vi "Node Archive and FTP File Handler ver2.vi"() -> ()   [LabVIEW 2010]
doc: "NODE ARCHIVE & FTP is a software used to handle the file management of remote field sites using the HTI Data Logger or ATR series acoustic equipment that generates *.RAT and *.ATL files. The software monitors a specific folder on the local machine that the HTI equipment has been set up to move completed files of these types into. All other file types are ignored. The software continues to scan this file until a new file is added to the directory, on the addition of a file the NODE ARCHIVE & FTP software moves the file into an Archive directory (and if specified into a redundant Archive directory) then creates a *.ZIP version of the file and retains a copy of it in the Archive directory as well. All Zip files are then copied to a specified FTP host.\n\nNODE ARCHIVE & FTP will not try and move files for the last five minutes of an hour, or for the first five to ten minutes of the hour (based on CPU time). This is to allow the HTI hardware time to move all files at the top of the hour and avoid conflict. During the rest of the hour the software will continue to scan for new files. At any time a user can force a scan or FTP move by selecting the Manual Force FTP button or the Manual Archive Files button.\n\nNODE ARCHIVE & FTP creates an .INI file and a .CSV file in the programs application directory. The .INI file retains the last values of the file directory and FTP credentials used. The .CSV retains a history of *.ZIP files moved to the FTP and the status of their move, if there were errors or not. NODE ARCHIVE & FTP will continue to try and send the file to the FTP host until that file has completed the process with no errors. DO NOT remove or edit the .CSV file or the software will try and move all files up to the FTP again and will slow down the FTP Host."
uses:
  FTP Credintials.ctl
  <vilib>/Utility/sysdir.llb/System Directory Type.ctl
  <vilib>/Utility/error.llb/DialogType.ctl
  <vilib>/Utility/config.llb/Read Key (String).vi
  <vilib>/Utility/config.llb/Read Key (Boolean).vi
  <vilib>/Utility/config.llb/Read Key (Path).vi
  <vilib>/Utility/config.llb/Read Key (I32).vi
  <vilib>/Utility/config.llb/Write Key (Path).vi
  <vilib>/Utility/config.llb/Write Key (String).vi
  <vilib>/Utility/config.llb/Write Key (I32).vi
  <vilib>/Utility/config.llb/Write Key (Boolean).vi
  <vilib>/Utility/config.llb/NI_LVConfig.lvlib
  Aarons labview builds/telemetryCode/Utilities/NewNI_SMTPEmail Folder/NewNI_SMTPEmail.lvlib
panel:
  in  "Time DaY":timestamp
  in  "Top level Tabs":T1(tab)
  in  "ShutDown":bool
  out "Status File move":bool caption="Archiving"
  out "Status FTP move":bool caption="FTP In Progress"
  in  "Manual FTP":bool
  in  "Manual Archive":bool
  in  "FTP Creds":T2 {"FTP Timeout (S)" min=0 max=300 step=1}
  in  "Archive Location 2":path caption="(Optional) External Directory To Archive *.RAT files"
  in  "Archive Location":path=path "C:/Archive" caption="Directory To Archive *.RAT files"
  in  "Rats Location":path=path "C:/Incoming" caption="Directory To Find *.RAT files"
  in  "Ping FTP Host":bool=TRUE
  in  "Ping Node 2":bool=TRUE
  in  "Ping Node 1":bool=TRUE
  out "Node 2 Response":bool
  in  "AddressNode2":string="www.google.com" caption="Address of Node 2 to Ping"
  out "FTP Response":bool
  out "Node1 Response":bool
  in  "recipients":string[](array[string])=["nmswyers@gmail.com"] caption="Email Recipients"
  in  "Addresshost":string="50.6.185.144" caption="Address of FTP host to Ping"
  in  "AddressNode 1":string="www.google.com" caption="Address of Node 1 to Ping"
  out "Elapsed Time (H)":dbl caption="Time to Next File \nSize Check (H)" format="%#_3f"
  out "Email Notification":T3 caption="Email Notification (From INI File)"
  # "DIRECTORY SETUP:"
  # "FTP SETUP:"
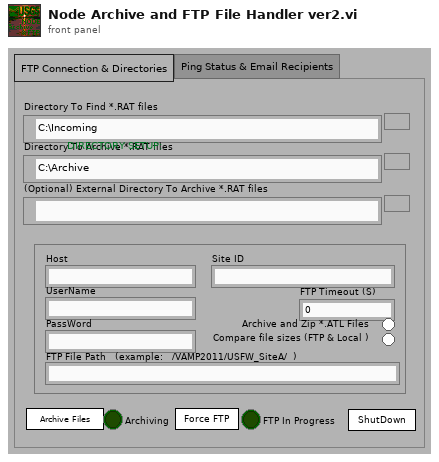
[diagram p1: front panel]
types:
  T1 = enum32{"FTP Connection & Directories", "Ping Status & Email Recipients"}
  T2 = typedef "FTP Credintials.ctl" = cluster{"Host":string, "UserName":string, "PassWord":string, "FTP File Path":string, "FTP Timeout (S)":i32, "Use ATL":bool, "Comp File Size":bool, "SITE ID":string, "Active or Passive":bool, "ASCII or Binary":bool}
  T3 = cluster{"Mail Server":string, "Return Address":string, "User Name":string, "Password":string}
  T4 = typedef "System Directory Type.ctl" = i32
  T5 = cluster{"Mail Server":string, "Return Address":string, "Email User Name":string, "Password":string}
  T6 = typedef "NI_LVConfig.lvlib/Config Data RefNum.ctl" = refnum<k1>
  T7 = typedef "DialogType.ctl" = u16
  T8 = cluster{"AddressNode 1":string, "AddressNode2":string, "Addresshost":string}
  T9 = enum16{"open", "replace", "create", "open or create", "replace or create", "replace or create with confirmation"}
  T10 = enum32{"invalid app kind", "Development System", "Run Time System", "Student Edition", "Embedded LabVIEW", "Evaluation", "Custom"}
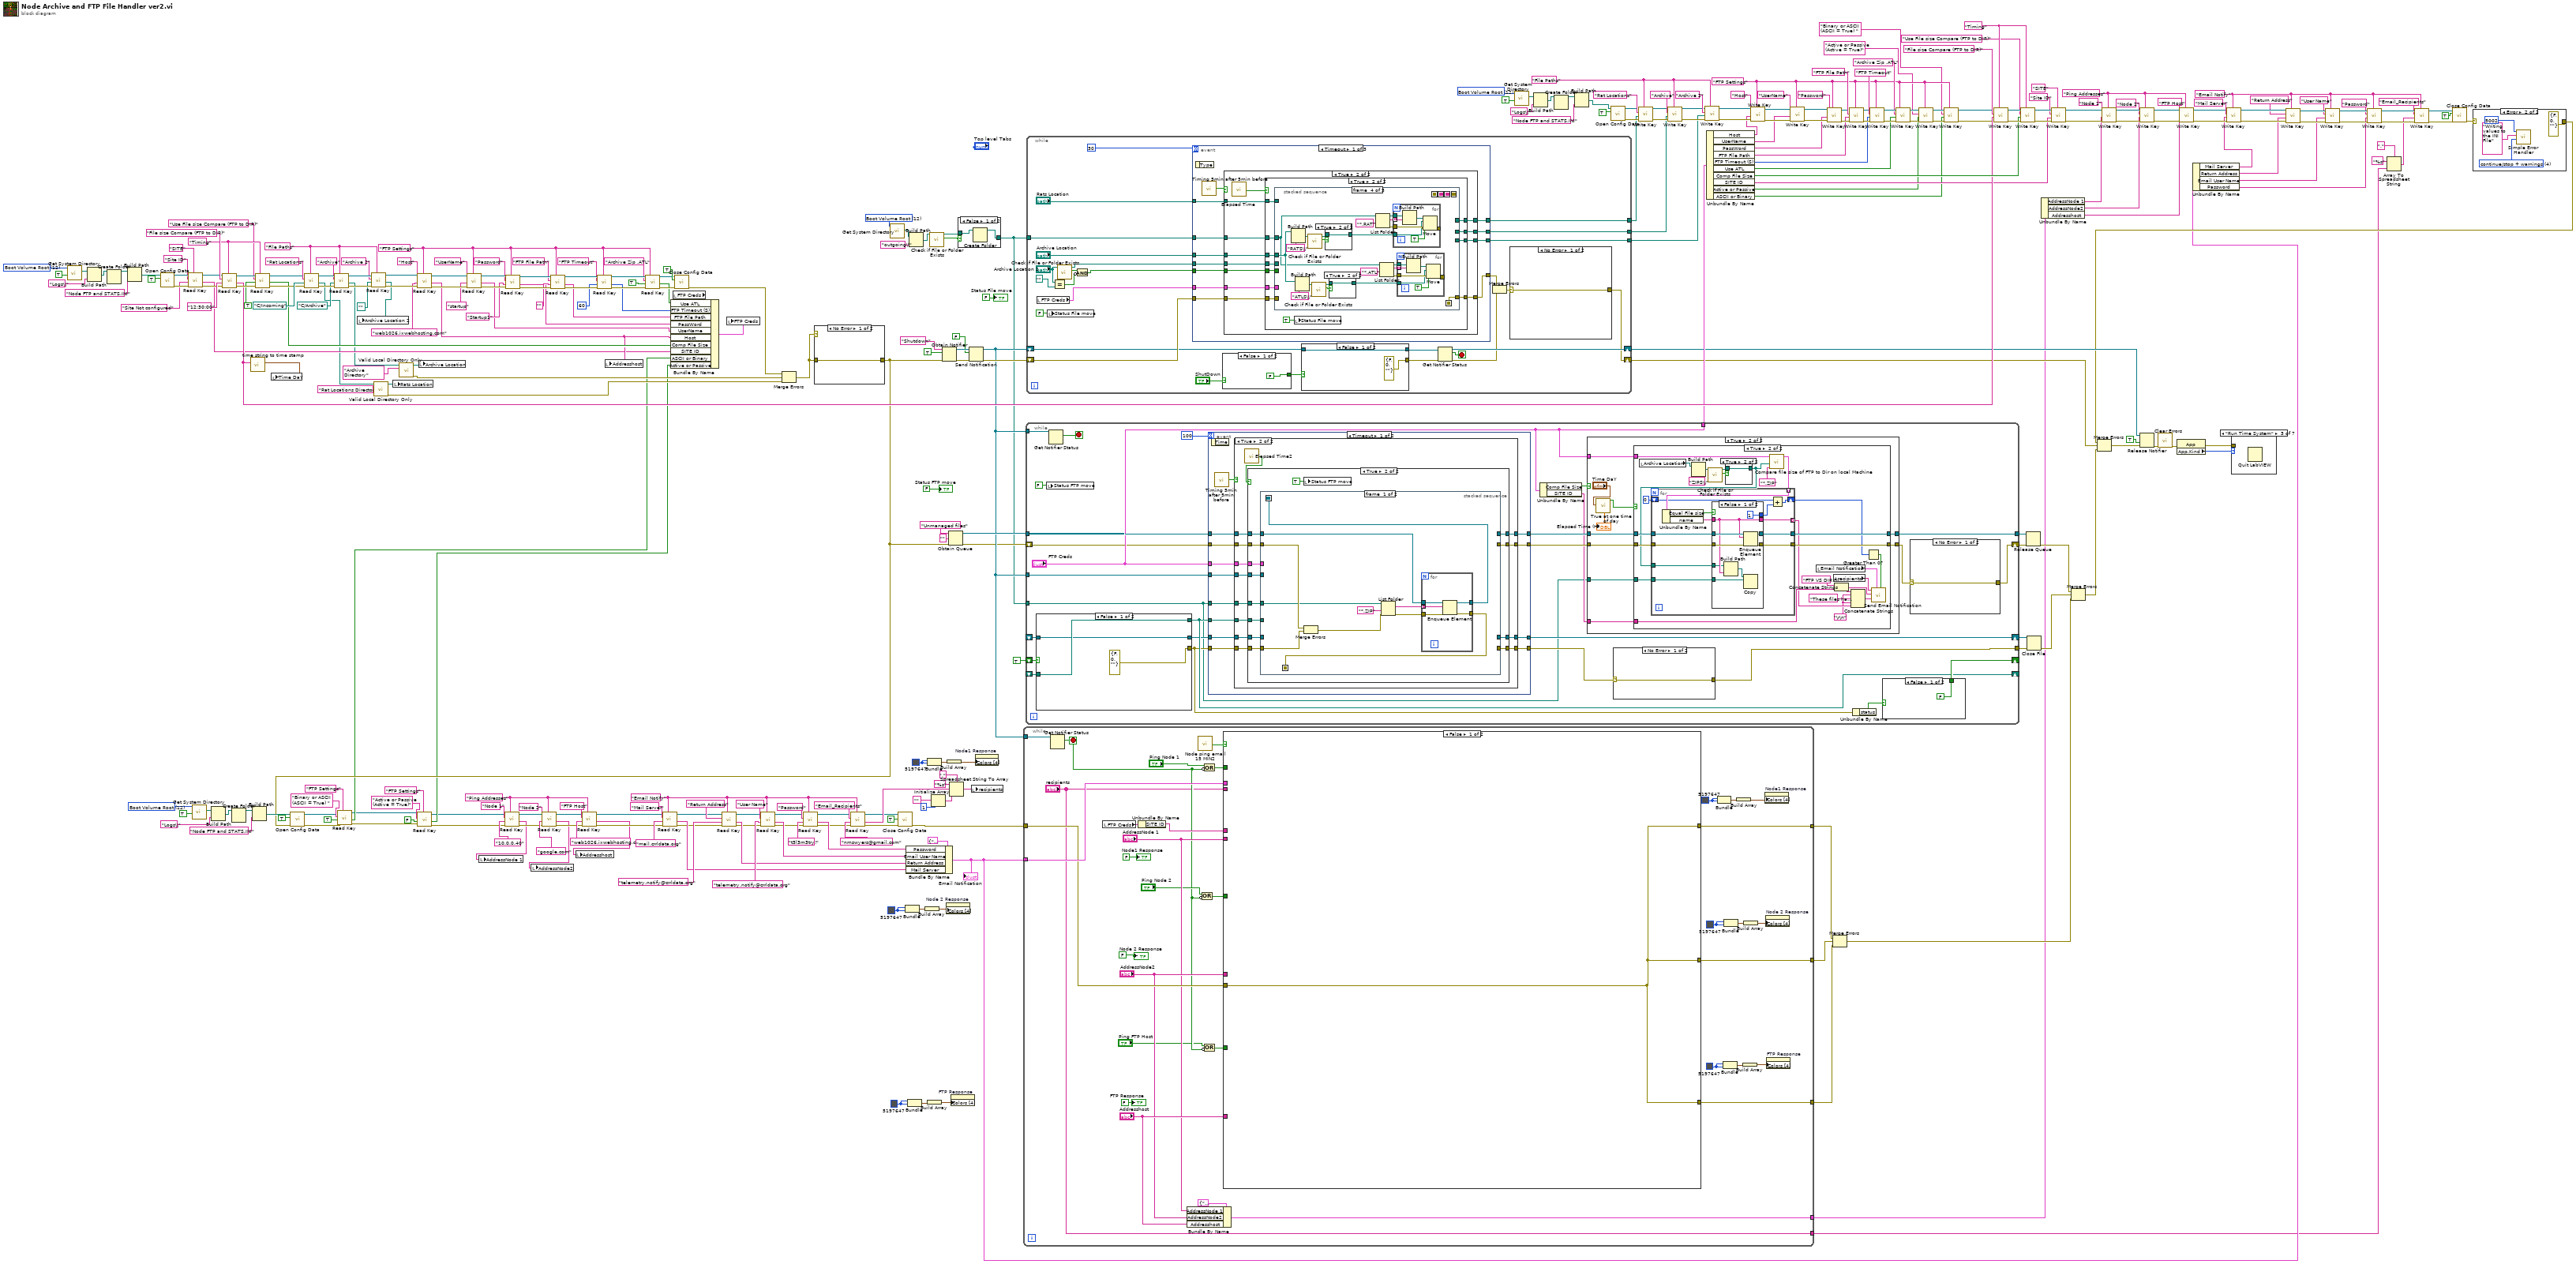
[diagram p0: block diagram]
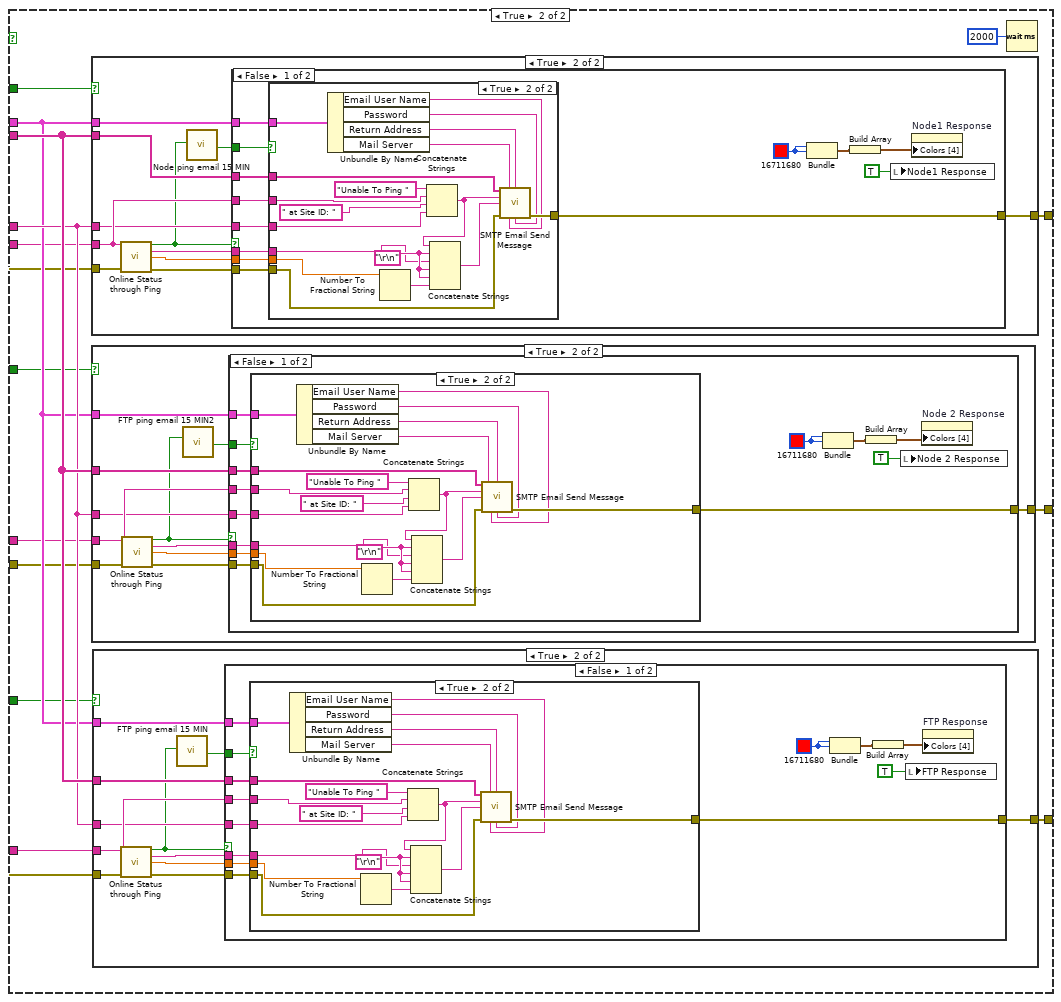
[diagram p3: hidden frame]
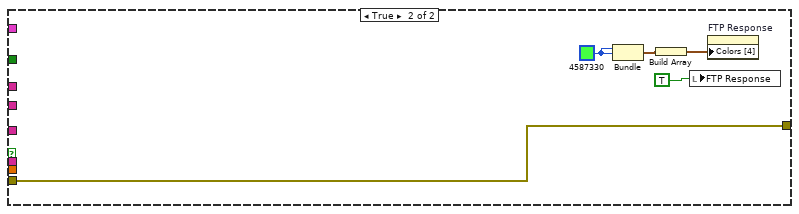
[diagram p6: hidden frame]
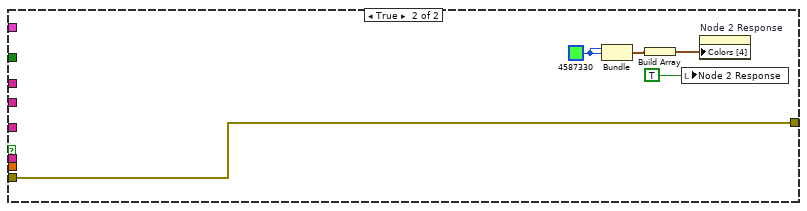
[diagram p9: hidden frame]
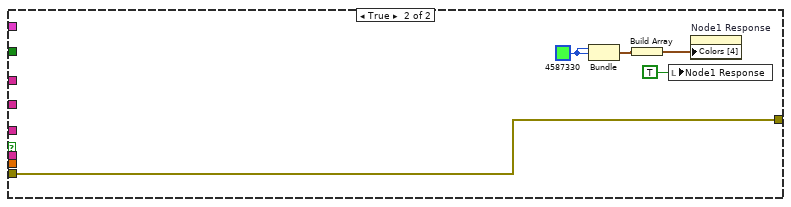
[diagram p12: hidden frame]
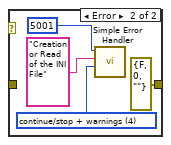
[diagram p14: hidden frame]
diagram:
  w21 = T4 12 items=["User Home"=0, "User Desktop"=1, "User Documents"=2, "User Application Data"=3, "User Preferences"=4, "User Temporary"=5, "Public Documents"=6, "Public Application Data"=7, "Public Preferences"=8, "Public Cache"=13, "System Core Libraries"=9, "System Installed Libraries"=10, "Application Files"=11, "Boot Volume Root"=12] ("system directory type")
  w26 = "Email Notify" ("name or relative path")
  w94 = "Ping Addresses" ("name or relative path")
  w107 = "Ping Addresses" ("name or relative path")
  w143 = u32 5197647 ("Color Box")
  w25 = "Email Notify" ("name or relative path")
  w153 = T4 12 items=["User Home"=0, "User Desktop"=1, "User Documents"=2, "User Application Data"=3, "User Preferences"=4, "User Temporary"=5, "Public Documents"=6, "Public Application Data"=7, "Public Preferences"=8, "Public Cache"=13, "System Core Libraries"=9, "System Installed Libraries"=10, "Application Files"=11, "Boot Volume Root"=12] ("system directory type")
  w169 = T4 12 items=["User Home"=0, "User Desktop"=1, "User Documents"=2, "User Application Data"=3, "User Preferences"=4, "User Temporary"=5, "Public Documents"=6, "Public Application Data"=7, "Public Preferences"=8, "Public Cache"=13, "System Core Libraries"=9, "System Installed Libraries"=10, "Application Files"=11, "Boot Volume Root"=12] ("system directory type")
  w207 = u32 5197647 ("Color Box")
  w204 = u32 5197647 ("Color Box")
  w215 = "Timing" ("name or relative path")
  w223 = "Timing" ("name or relative path")
  w7 = "FTP Settings" ("name or relative path")
  w262 = "File Paths" ("name or relative path")
  w297 = "FTP Settings" ("name or relative path")
  w315 = "File Paths" ("name or relative path")
  w317 = T4 12 items=["User Home"=0, "User Desktop"=1, "User Documents"=2, "User Application Data"=3, "User Preferences"=4, "User Temporary"=5, "Public Documents"=6, "Public Application Data"=7, "Public Preferences"=8, "Public Cache"=13, "System Core Libraries"=9, "System Installed Libraries"=10, "Application Files"=11, "Boot Volume Root"=12] ("system directory type")
  n1 = call <vilib>:"Get System Directory.vi"("create directory if not found? (F)"=TRUE, "system directory type"=w317) -> ("system directory"=w318:path)  [unwired: 9 in]
  n2 = Build Path(base path=w318, name or relative path="Logs\\" ("string")) -> (appended path=w179:path)
  n3 = Create Folder(path (use dialog)=w179) -> (created path=w178:path)  [unwired: 2 in, 2 out]
  n4 = Build Path(base path=w178, name or relative path="Node FTP and STATS.INI") -> (appended path=w176:path)
  n5 = call <vilib>:"Open Config Data.vi"("create file if necessary (T)"=TRUE, "configuration file path"=w176) -> ("error out"=w202:errorcluster, "refnum"=w201:T6)  [unwired: 7 in, 1 out]
  n6 = call-poly <vilib>:"Read Key.vi"("section"="SITE" ("name or relative path"), "error in (no error)"=w202, "default value"="Site Not configured", "key"="Site ID" ("name or relative path"), "refnum"=w201) -> ("error out"=w199:errorcluster, "value"=w195:string, "refnum out"=w200:T6)  [unwired: 3 in, 1 out]
  n7 = call <vilib>:"Get System Directory.vi"("create directory if not found? (F)"=TRUE, "system directory type"=w153) -> ("system directory"=w152:path)  [unwired: 9 in]
  n8 = Build Path(base path=w152, name or relative path="Logs\\" ("string")) -> (appended path=w158:path)
  n9 = call-poly <vilib>:"Read Key.vi"("section"=w223, "error in (no error)"=w199, "default value"="12:30:00", "key"="File size Compare (FTP to DIR)" ("name or relative path"), "refnum"=w200) -> ("error out"=w227:errorcluster, "value"=w210:string, "refnum out"=w226:T6)  [unwired: 3 in, 1 out]
  n10 = Create Folder(path (use dialog)=w158) -> (created path=w159:path)  [unwired: 2 in, 2 out]
  n11 = call "time string to time stamp.vi"("time string example(16:15:00)"=w210) -> ("time stamp"=w220:timestamp)  [unwired: 10 in]
  n12 = Build Path(base path=w159, name or relative path="Node FTP and STATS.INI") -> (appended path=w161:path)
  n13 = call-poly <vilib>:"Read Key.vi"("section"=w223, "error in (no error)"=w227, "default value"=TRUE ("create file if necessary (T)"), "key"="Use File size Compare (FTP to DIR)" ("name or relative path"), "refnum"=w226) -> ("error out"=w224:errorcluster, "value"=w212:bool, "refnum out"=w225:T6)  [unwired: 3 in, 1 out]
  n14 = local write "Time DaY"(w220) -> ()
  n15 = call-poly <vilib>:"Read Key.vi"("section"=w315, "error in (no error)"=w224, "default value"=path "C:/Incoming", "key"="Rat Locations" ("name or relative path"), "refnum"=w225) -> ("error out"=w322:errorcluster, "value"=w188:path, "refnum out"=w323:T6)  [unwired: 3 in, 1 out]
  n16 = call-poly <vilib>:"Read Key.vi"("section"=w315, "error in (no error)"=w322, "default value"=path "C:/Archive", "key"="Archive" ("name or relative path"), "refnum"=w323) -> ("error out"=w320:errorcluster, "value"=w184:path, "refnum out"=w321:T6)  [unwired: 3 in, 1 out]
  n17 = call-poly <vilib>:"Read Key.vi"("section"=w315, "error in (no error)"=w320, "default value"=path "", "key"="Archive 2" ("name or relative path"), "refnum"=w321) -> ("error out"=w311:errorcluster, "value"=w175:path, "refnum out"=w304:T6)  [unwired: 3 in, 1 out]
  n18 = local write "Archive Location 2"(w175) -> ()
  n19 = call "Valid Local Directory Only.vi"("Directory ref"="Rat Locations Directory", "Path input"=w188) -> ("error out"=w163:errorcluster, "Path output"=w186:path)  [unwired: 8 in]
  n20 = local write "Rats Location"(w186) -> ()
  n21 = call "Valid Local Directory Only.vi"("Directory ref"="Archive Directory", "Path input"=w184) -> ("error out"=w164:errorcluster, "Path output"=w183:path)  [unwired: 8 in]
  n22 = call-poly <vilib>:"Read Key.vi"("section"=w297, "error in (no error)"=w311, "default value"="web1026.ixwebhosting.com" ("name or relative path"), "key"="Host" ("name or relative path"), "refnum"=w304) -> ("error out"=w310:errorcluster, "value"=w208:string, "refnum out"=w303:T6)  [unwired: 3 in, 1 out]
  n23 = local write "Archive Location"(w183) -> ()
  n24 = call-poly <vilib>:"Read Key.vi"("section"=w297, "error in (no error)"=w310, "default value"="startup" ("name or relative path"), "key"="UserName" ("name or relative path"), "refnum"=w303) -> ("error out"=w309:errorcluster, "value"=w242:string, "refnum out"=w302:T6)  [unwired: 3 in, 1 out]
  n25 = call-poly <vilib>:"Read Key.vi"("section"=w297, "error in (no error)"=w309, "default value"="Startup1" ("name or relative path"), "key"="Password" ("name or relative path"), "refnum"=w302) -> ("error out"=w308:errorcluster, "value"=w243:string, "refnum out"=w301:T6)  [unwired: 3 in, 1 out]
  n26 = call-poly <vilib>:"Read Key.vi"("section"=w297, "error in (no error)"=w308, "default value"="" ("name or relative path"), "key"="FTP File Path" ("name or relative path"), "refnum"=w301) -> ("error out"=w307:errorcluster, "value"=w244:string, "refnum out"=w300:T6)  [unwired: 3 in, 1 out]
  n27 = call-poly <vilib>:"Read Key.vi"("section"=w297, "error in (no error)"=w307, "default value"=60, "key"="FTP Timeout" ("name or relative path"), "refnum"=w300) -> ("error out"=w306:errorcluster, "value"=w81:i32, "refnum out"=w299:T6)  [unwired: 3 in, 1 out]
  n28 = local write "Addresshost"(w208) -> ()
  n29 = call-poly <vilib>:"Read Key.vi"("section"=w297, "error in (no error)"=w306, "default value"=TRUE, "key"="Archive Zip .ATL" ("name or relative path"), "refnum"=w299) -> ("error out"=w305:errorcluster, "value"=w245:bool, "refnum out"=w298:T6)  [unwired: 3 in, 1 out]
  n30 = local read "FTP Creds"() -> (w246:T2)
  n31 = call <vilib>:"Close Config Data.vi"("error in (no error)"=w305, "write file if changed (T)"=TRUE, "refnum"=w298) -> ("error out"=w165:errorcluster)  [unwired: 7 in, 1 out]
  n32 = Merge Errors(w165, w164, w163) -> (w166:errorcluster)
  n33 = case shown="No Error" w166 {
    tunnel: w166 -> [w325 _]
    tunnel: [w325 errorcluster {"status"=FALSE, "code"=0, "source"=""} ("error out")] -> w118
    frame No Error {
    }
    frame Error {
      w329 = T7 4 items=["no dialog", "OK message", "continue or stop message", "OK message + warnings", "continue/stop + warnings"] ("type of dialog (OK msg:1)")
      n34 = call <vilib>:"Simple Error Handler.vi"("error code (no error:0)"=5001, "error source (\" \")"="Creation or Read of the INI File" ("error source (\" \")"), "type of dialog (OK msg:1)"=w329) -> ()  [unwired: 2 in, 5 out]
    }
  }
  n35 = call <vilib>:"Open Config Data.vi"("error in (no error)"=w118, "create file if necessary (T)"=TRUE, "configuration file path"=w161) -> ("error out"=w73:errorcluster, "refnum"=w74:T6)  [unwired: 6 in, 1 out]
  n36 = call-poly <vilib>:"Read Key.vi"("section"="FTP Settings" ("name or relative path"), "error in (no error)"=w73, "default value"=TRUE, "key"="Binary or ASCII (ASCII = True) " ("name or relative path"), "refnum"=w74) -> ("error out"=w14:errorcluster, "value"=w17:bool, "refnum out"=w15:T6)  [unwired: 3 in, 1 out]
  n37 = call-poly <vilib>:"Read Key.vi"("section"="FTP Settings" ("name or relative path"), "error in (no error)"=w14, "default value"=FALSE, "key"="Active or Passive (Active = True)" ("name or relative path"), "refnum"=w15) -> ("error out"=w12:errorcluster, "value"=w16:bool, "refnum out"=w13:T6)  [unwired: 3 in, 1 out]
  n38 = call-poly <vilib>:"Read Key.vi"("section"=w107, "error in (no error)"=w12, "default value"="10.0.0.40", "key"="Node 1" ("Mail Server"), "refnum"=w13) -> ("error out"=w105:errorcluster, "value"=w100:string, "refnum out"=w106:T6)  [unwired: 3 in, 1 out]
  n39 = local write "AddressNode 1"(w100) -> ()
  n40 = call-poly <vilib>:"Read Key.vi"("section"=w107, "error in (no error)"=w105, "default value"="google.com", "key"="Node 2" ("Mail Server"), "refnum"=w106) -> ("error out"=w104:errorcluster, "value"=w99:string, "refnum out"=w103:T6)  [unwired: 3 in, 1 out]
  n41 = local write "AddressNode2"(w99) -> ()
  n42 = call-poly <vilib>:"Read Key.vi"("section"=w107, "error in (no error)"=w104, "default value"="web1026.ixwebhosting.com", "key"="FTP Host" ("Mail Server"), "refnum"=w103) -> ("error out"=w101:errorcluster, "value"=w98:string, "refnum out"=w102:T6)  [unwired: 3 in, 1 out]
  n43 = local write "Addresshost"(w98) -> ()
  n44 = call-poly <vilib>:"Read Key.vi"("section"=w25, "error in (no error)"=w101, "default value"="mail.crrldata.org", "key"="Mail Server" ("Mail Server"), "refnum"=w102) -> ("error out"=w71:errorcluster, "value"=w132:string, "refnum out"=w70:T6)  [unwired: 3 in, 1 out]
  n45 = Bundle By Name(cluster=w246, "Use ATL"=w245, "FTP Timeout (S)"=w81, "FTP File Path"=w244, "PassWord"=w243, "UserName"=w242, "Host"=w208, "Comp File Size"=w212, "SITE ID"=w195, "ASCII or Binary"=w17, "Active or Passive"=w16) -> (w247:T2)
  n46 = call-poly <vilib>:"Read Key.vi"("section"=w25, "error in (no error)"=w71, "default value"="telemetry.notify@crrldata.org", "key"="Return Address" ("Return Address"), "refnum"=w70) -> ("error out"=w69:errorcluster, "value"=w133:string, "refnum out"=w66:T6)  [unwired: 3 in, 1 out]
  n47 = local write "FTP Creds"(w247) -> ()
  n48 = call-poly <vilib>:"Read Key.vi"("section"=w25, "error in (no error)"=w69, "default value"="telemetry.notify@crrldata.org", "key"="User Name" ("Email User Name"), "refnum"=w66) -> ("error out"=w68:errorcluster, "value"=w134:string, "refnum out"=w67:T6)  [unwired: 3 in, 1 out]
  n49 = call-poly <vilib>:"Read Key.vi"("section"=w25, "error in (no error)"=w68, "default value"="t3l3m3try!", "key"="Password" ("Password"), "refnum"=w67) -> ("error out"=w57:errorcluster, "value"=w135:string, "refnum out"=w58:T6)  [unwired: 3 in, 1 out]
  n50 = call-poly <vilib>:"Read Key.vi"("section"=w25, "error in (no error)"=w57, "default value"="nmswyers@gmail.com", "key"="Email_Recipients" ("Password"), "refnum"=w58) -> ("error out"=w54:errorcluster, "value"=w56:string, "refnum out"=w55:T6)  [unwired: 3 in, 1 out]
  n51 = call <vilib>:"Get System Directory.vi"("system directory type"=w21) -> ("system directory"=w22:path)  [unwired: 10 in]
  n52 = call <vilib>:"Close Config Data.vi"("error in (no error)"=w54, "write file if changed (T)"=TRUE, "refnum"=w55) -> ("error out"=w146:errorcluster)  [unwired: 7 in, 1 out]
  n53 = Bundle("Color Box"=w207, "Color Box"=w207) -> (w206:cluster{"Color Box":u32, "Color Box":u32})  [unwired: 1 in]
  n54 = Bundle By Name(cluster=T5 {"Mail Server"="Mail Server", "Return Address"="Return Address", "Email User Name"="User Name", "Password"="Password"} ("input cluster"), "Password"=w135, "Email User Name"=w134, "Return Address"=w133, "Mail Server"=w132) -> (w35:T5)
  "Email Notification" <- w35
  n55 = Bundle("Color Box"=w143, "Color Box"=w143) -> (w144:cluster{"Color Box":u32, "Color Box":u32})  [unwired: 1 in]
  n56 = Build Path(base path=w22, name or relative path="outgoing\\") -> (appended path=w19:path)
  n57 = Build Array(w206) -> (w142:cluster{"Color Box":u32, "Color Box":u32}[])
  n58 = Bundle("Color Box"=w204, "Color Box"=w204) -> (w203:cluster{"Color Box":u32, "Color Box":u32})  [unwired: 1 in]
  n59 = Build Array(w144) -> (w145:cluster{"Color Box":u32, "Color Box":u32}[])
  n60 = call <vilib>:"Check if File or Folder Exists.vi"("path"=w19) -> ("file or folder exists?"=w23:bool, "dup path"=w24:path)  [unwired: 8 in, 1 out]
  n61 = Initialize Array("", 1 ("dimension size")) -> (w65:string[])
  n62 = Obtain Notifier(name (unnamed)="Shutdown", notification data type=TRUE, error in (no error)=w118) -> (notifier out=w129:refnum<notifier>, error out=w127:errorcluster)  [unwired: 1 in, 1 out]
  n63 = property on="Node 2 Response" class="Bool (strict)"("Colors [4]"=w142) -> ()  [unwired: 2 in, 2 out]
  n64 = Build Array(w203) -> (w205:cluster{"Color Box":u32, "Color Box":u32}[])
  n65 = Obtain Queue(name (unnamed)="Unmanaged files", element data type="" ("name (unnamed)"), error in (no error)=w118) -> (queue out=w234:refnum<queue>, error out=w72:errorcluster)  [unwired: 2 in, 1 out]
  n66 = Spreadsheet String To Array(delimiter (Tab)=",", format string="%s", spreadsheet string=w56, array type (2D Dbl)=w65) -> (array=w53:string[])
  n67 = property on="FTP Response" class="Bool (strict)"("Colors [4]"=w145) -> ()  [unwired: 2 in, 2 out]
  n68 = case shown="False" w23 {
    tunnel: w24 -> [w331 w332]
    tunnel: [w330 w332] -> w18
    frame False {
      n69 = Create Folder(path (use dialog)=w331) -> (created path=w330:path)  [unwired: 2 in, 2 out]
    }
    frame True {
    }
  }
  n70 = Send Notification(notification=FALSE, notifier=w129, error in (no error)=w127) -> (notifier out=w82:refnum<notifier>, error out=w126:errorcluster)
  n71 = local write "recipients"(w53) -> ()
  n72 = property on="Node1 Response" class="Bool (strict)"("Colors [4]"=w205) -> ()  [unwired: 2 in, 2 out]
  n73 = while {
    tunnel: w146 -> [w356]
    tunnel: [w363] -> w182
    tunnel: w35 -> [w358]
    tunnel: [w360] -> w141
    tunnel: [w359] -> w140
    tunnel: w82 -> [w357]
    tunnel: [w351] -> w97
    tunnel: ["recipients"] -> w30
    stop <- w345 stop-if-true
    w337 = u32 5197647 ("Color Box")
    w338 = u32 5197647 ("Color Box")
    w342 = u32 5197647 ("Color Box")
    n74 = Get Notifier Status(notifier=w357) -> (current notification=w345:bool)  [unwired: 1 in, 4 out]
    n75 = local read "FTP Creds"() -> (w364:T2)
    n76 = Unbundle By Name(w364) -> ("SITE ID"=w361:string)
    n77 = Bundle By Name(cluster=T8 {"AddressNode 1"="www.google.com", "AddressNode2"="www.google.com", "Addresshost"="50.6.185.144"} ("input cluster"), "AddressNode 1"="AddressNode 1", "AddressNode2"="AddressNode2", "Addresshost"="Addresshost") -> (w351:T8)
    n78 = call "Node ping email 15 MIN2"() -> ("Time has Elapsed"=w334:bool)  [unwired: 12 in, 7 out]
    n79 = Compound Arithmetic op=OR("Ping Node 2", invert w345) -> (w348:bool)
    n80 = Compound Arithmetic op=OR("Ping Node 1", invert w345) -> (w350:bool)
    n81 = Compound Arithmetic op=OR("Ping FTP Host", invert w345) -> (w346:bool)
    n82 = case shown="False" w334 {
      tunnel: [w367 w381] -> w363
      tunnel: "recipients" -> [_ w380]
      tunnel: w361 -> [_ w379]
      tunnel: [w367 w378] -> w360
      tunnel: [w367 w377] -> w359
      tunnel: w358 -> [_ w376]
      tunnel: w356 -> [w367 w375]
      tunnel: "Addresshost" -> [_ w374]
      tunnel: "AddressNode2" -> [_ w373]
      tunnel: "AddressNode 1" -> [_ w372]
      tunnel: w350 -> [_ w371]
      tunnel: w348 -> [_ w370]
      tunnel: w346 -> [_ w369]
      frame False {
      }
      frame True {
        n83 = case shown="True" w371 {
          tunnel: w372 -> [_ w489]
          tunnel: [w480 w487] -> w381
          tunnel: w380 -> [_ w486]
          tunnel: w375 -> [w480 w485]
          tunnel: w379 -> [_ w484]
          tunnel: w376 -> [_ w483]
          frame False {
          }
          frame True {
            n84 = call "Online Status through Ping.vi"("AddressToPing"=w489, "error in (no error)"=w485) -> ("Connection?"=w481:bool, "Standard Output"=w491:string, "% Recieved"=w490:dbl, "error out"=w488:errorcluster)  [unwired: 9 in, 1 out]
            n85 = call "Node ping email 15 MIN"("Reset"=w481) -> ("Time has Elapsed"=w482:bool)  [unwired: 11 in, 7 out]
            n86 = case shown="False" w481 {
              tunnel: w491 -> [w504 _]
              tunnel: w490 -> [w503 _]
              tunnel: w486 -> [w502 _]
              tunnel: w489 -> [w501 _]
              tunnel: w484 -> [w496 _]
              tunnel: w488 -> [w495 w524]
              tunnel: [w494 w524] -> w487
              tunnel: w483 -> [w493 _]
              tunnel: w482 -> [w492 _]
              frame False {
                w499 = u32 16711680 ("Color Box")
                n87 = case shown="True" w492 {
                  tunnel: w504 -> [_ w515]
                  tunnel: w503 -> [_ w518]
                  tunnel: w502 -> [_ w517]
                  tunnel: w501 -> [_ w516]
                  tunnel: w496 -> [_ w513]
                  tunnel: w495 -> [w505 w512]
                  tunnel: [w505 w511] -> w494
                  tunnel: w493 -> [_ w510]
                  frame False {
                  }
                  frame True {
                    w522 = "\r\n"
                    n88 = Unbundle By Name(w510) -> ("Email User Name"=w506:string, "Password"=w507:string, "Return Address"=w508:string, "Mail Server"=w509:string)
                    n89 = Number To Fractional String(number=w518) -> (F-format string=w521:string)  [unwired: 3 in]
                    n90 = Concatenate Strings("Unable To Ping " ("subject ([No Subject])"), w516, " at Site ID: " ("string"), w513) -> (w520:string)
                    n91 = Concatenate Strings(w520, w522, w515, w522, w522, w521) -> (w519:string)
                    n92 = call "SMTP Email Send Message.vi"("recipients"=w517, "mail server"=w509, "return address"=w508, "subject ([No Subject])"=w520, "message"=w519, "error in (no error)"=w512, "username"=w506, "password"=w507) -> ("error out"=w511:errorcluster)  [unwired: 7 out]
                  }
                }
                n93 = Bundle("Color Box"=w499, "Color Box"=w499) -> (w498:cluster{"Color Box":u32, "Color Box":u32})  [unwired: 1 in]
                n94 = Build Array(w498) -> (w500:cluster{"Color Box":u32, "Color Box":u32}[])
                n95 = local write "Node1 Response"(TRUE ("Node Responding")) -> ()
                n96 = property on="Node1 Response" class="Bool (strict)"("Colors [4]"=w500) -> ()  [unwired: 2 in, 2 out]
              }
              frame True {
                w527 = u32 4587330 ("Color Box")
                n97 = Bundle("Color Box"=w527, "Color Box"=w527) -> (w528:cluster{"Color Box":u32, "Color Box":u32})  [unwired: 1 in]
                n98 = Build Array(w528) -> (w526:cluster{"Color Box":u32, "Color Box":u32}[])
                n99 = local write "Node1 Response"(TRUE ("Node Responding")) -> ()
                n100 = property on="Node1 Response" class="Bool (strict)"("Colors [4]"=w526) -> ()  [unwired: 2 in, 2 out]
              }
            }
          }
        }
        n101 = case shown="True" w370 {
          tunnel: w373 -> [_ w439]
          tunnel: w380 -> [_ w438]
          tunnel: w375 -> [w431 w437]
          tunnel: w379 -> [_ w436]
          tunnel: [w431 w435] -> w378
          tunnel: w376 -> [_ w434]
          frame False {
          }
          frame True {
            n102 = call "Online Status through Ping.vi"("AddressToPing"=w439, "error in (no error)"=w437) -> ("Connection?"=w432:bool, "Standard Output"=w441:string, "% Recieved"=w440:dbl, "error out"=w442:errorcluster)  [unwired: 9 in, 1 out]
            n103 = call "FTP ping email 15 MIN2"("Reset"=w432) -> ("Time has Elapsed"=w433:bool)  [unwired: 11 in, 7 out]
            n104 = case shown="False" w432 {
              tunnel: w441 -> [w455 _]
              tunnel: w440 -> [w454 _]
              tunnel: w438 -> [w453 _]
              tunnel: w439 -> [w452 _]
              tunnel: w436 -> [w449 _]
              tunnel: w442 -> [w448 w477]
              tunnel: [w447 w477] -> w435
              tunnel: w434 -> [w444 _]
              tunnel: w433 -> [w443 _]
              frame False {
                w451 = u32 16711680 ("Color Box")
                n105 = case shown="True" w443 {
                  tunnel: w455 -> [_ w466]
                  tunnel: w454 -> [_ w469]
                  tunnel: w453 -> [_ w468]
                  tunnel: w452 -> [_ w467]
                  tunnel: w449 -> [_ w464]
                  tunnel: w448 -> [w456 w463]
                  tunnel: [w456 w462] -> w447
                  tunnel: w444 -> [_ w461]
                  frame False {
                  }
                  frame True {
                    w473 = "\r\n"
                    n106 = Unbundle By Name(w461) -> ("Email User Name"=w457:string, "Password"=w458:string, "Return Address"=w459:string, "Mail Server"=w460:string)
                    n107 = Number To Fractional String(number=w469) -> (F-format string=w472:string)  [unwired: 3 in]
                    n108 = Concatenate Strings("Unable To Ping " ("subject ([No Subject])"), w467, " at Site ID: " ("string"), w464) -> (w471:string)
                    n109 = Concatenate Strings(w471, w473, w466, w473, w473, w472) -> (w470:string)
                    n110 = call "SMTP Email Send Message.vi"("recipients"=w468, "mail server"=w460, "return address"=w459, "subject ([No Subject])"=w471, "message"=w470, "error in (no error)"=w463, "username"=w457, "password"=w458) -> ("error out"=w462:errorcluster)  [unwired: 7 out]
                  }
                }
                n111 = Bundle("Color Box"=w451, "Color Box"=w451) -> (w450:cluster{"Color Box":u32, "Color Box":u32})  [unwired: 1 in]
                n112 = Build Array(w450) -> (w446:cluster{"Color Box":u32, "Color Box":u32}[])
                n113 = local write "Node 2 Response"(TRUE ("FTP Responding")) -> ()
                n114 = property on="Node 2 Response" class="Bool (strict)"("Colors [4]"=w446) -> ()  [unwired: 2 in, 2 out]
              }
              frame True {
                w479 = u32 4587330 ("Color Box")
                n115 = Bundle("Color Box"=w479, "Color Box"=w479) -> (w478:cluster{"Color Box":u32, "Color Box":u32})  [unwired: 1 in]
                n116 = Build Array(w478) -> (w476:cluster{"Color Box":u32, "Color Box":u32}[])
                n117 = local write "Node 2 Response"(TRUE) -> ()
                n118 = property on="Node 2 Response" class="Bool (strict)"("Colors [4]"=w476) -> ()  [unwired: 2 in, 2 out]
              }
            }
          }
        }
        n119 = case shown="True" w369 {
          tunnel: w374 -> [_ w393]
          tunnel: w380 -> [_ w389]
          tunnel: w375 -> [w382 w388]
          tunnel: w379 -> [_ w387]
          tunnel: [w382 w386] -> w377
          tunnel: w376 -> [_ w385]
          frame False {
          }
          frame True {
            n120 = call "Online Status through Ping.vi"("AddressToPing"=w393, "error in (no error)"=w388) -> ("Connection?"=w383:bool, "Standard Output"=w391:string, "% Recieved"=w392:dbl, "error out"=w390:errorcluster)  [unwired: 9 in, 1 out]
            n121 = call "FTP ping email 15 MIN"("Reset"=w383) -> ("Time has Elapsed"=w384:bool)  [unwired: 11 in, 7 out]
            n122 = case shown="False" w383 {
              tunnel: w391 -> [w406 _]
              tunnel: w392 -> [w405 _]
              tunnel: w389 -> [w404 _]
              tunnel: w393 -> [w403 _]
              tunnel: w387 -> [w398 _]
              tunnel: w390 -> [w397 w426]
              tunnel: [w396 w426] -> w386
              tunnel: w385 -> [w395 _]
              tunnel: w384 -> [w394 _]
              frame False {
                w402 = u32 16711680 ("Color Box")
                n123 = case shown="True" w394 {
                  tunnel: w406 -> [_ w417]
                  tunnel: w405 -> [_ w420]
                  tunnel: w404 -> [_ w419]
                  tunnel: w403 -> [_ w418]
                  tunnel: w398 -> [_ w415]
                  tunnel: w397 -> [w407 w414]
                  tunnel: [w407 w413] -> w396
                  tunnel: w395 -> [_ w412]
                  frame False {
                  }
                  frame True {
                    w424 = "\r\n"
                    n124 = Unbundle By Name(w412) -> ("Email User Name"=w408:string, "Password"=w409:string, "Return Address"=w410:string, "Mail Server"=w411:string)
                    n125 = Number To Fractional String(number=w420) -> (F-format string=w423:string)  [unwired: 3 in]
                    n126 = Concatenate Strings("Unable To Ping " ("subject ([No Subject])"), w418, " at Site ID: " ("string"), w415) -> (w422:string)
                    n127 = Concatenate Strings(w422, w424, w417, w424, w424, w423) -> (w421:string)
                    n128 = call "SMTP Email Send Message.vi"("recipients"=w419, "mail server"=w411, "return address"=w410, "subject ([No Subject])"=w422, "message"=w421, "error in (no error)"=w414, "username"=w408, "password"=w409) -> ("error out"=w413:errorcluster)  [unwired: 7 out]
                  }
                }
                n129 = Bundle("Color Box"=w402, "Color Box"=w402) -> (w401:cluster{"Color Box":u32, "Color Box":u32})  [unwired: 1 in]
                n130 = Build Array(w401) -> (w400:cluster{"Color Box":u32, "Color Box":u32}[])
                n131 = local write "FTP Response"(TRUE ("FTP Responding")) -> ()
                n132 = property on="FTP Response" class="Bool (strict)"("Colors [4]"=w400) -> ()  [unwired: 2 in, 2 out]
              }
              frame True {
                w429 = u32 4587330 ("Color Box")
                n133 = Bundle("Color Box"=w429, "Color Box"=w429) -> (w428:cluster{"Color Box":u32, "Color Box":u32})  [unwired: 1 in]
                n134 = Build Array(w428) -> (w427:cluster{"Color Box":u32, "Color Box":u32}[])
                n135 = local write "FTP Response"(TRUE) -> ()
                n136 = property on="FTP Response" class="Bool (strict)"("Colors [4]"=w427) -> ()  [unwired: 2 in, 2 out]
              }
            }
          }
        }
        n137 = Wait (ms)(milliseconds to wait=u32 2000) -> ()  [unwired: 1 out]
      }
    }
    n138 = Bundle("Color Box"=w342, "Color Box"=w342) -> (w343:cluster{"Color Box":u32, "Color Box":u32})  [unwired: 1 in]
    n139 = Bundle("Color Box"=w338, "Color Box"=w338) -> (w339:cluster{"Color Box":u32, "Color Box":u32})  [unwired: 1 in]
    n140 = Bundle("Color Box"=w337, "Color Box"=w337) -> (w336:cluster{"Color Box":u32, "Color Box":u32})  [unwired: 1 in]
    n141 = Build Array(w343) -> (w341:cluster{"Color Box":u32, "Color Box":u32}[])
    n142 = Build Array(w339) -> (w340:cluster{"Color Box":u32, "Color Box":u32}[])
    n143 = Build Array(w336) -> (w335:cluster{"Color Box":u32, "Color Box":u32}[])
    n144 = property on="Node1 Response" class="Bool (strict)"("Colors [4]"=w341) -> ()  [unwired: 2 in, 2 out]
    n145 = property on="Node 2 Response" class="Bool (strict)"("Colors [4]"=w335) -> ()  [unwired: 2 in, 2 out]
    n146 = property on="FTP Response" class="Bool (strict)"("Colors [4]"=w340) -> ()  [unwired: 2 in, 2 out]
    "Node1 Response" <- FALSE
    "FTP Response" <- FALSE ("FTP Responding")
    "Node 2 Response" <- FALSE ("FTP Responding")
  }
  n147 = while {
    tunnel: w234 -> [w553]
    tunnel: [w544] -> w218
    shift-right: [w548] -> _
    shift-left: TRUE ("create directory if not found? (F)") -> [w551]
    shift-right: [w554] -> w237
    shift-left: _ -> [w550]
    shift-right: [w547] -> _
    shift-left: _ -> [w546]
    tunnel: ["FTP Creds"] -> w189
    tunnel: w82 -> [w537]
    tunnel: [w531] -> w114
    shift-right: [w535] -> w115
    shift-left: w72 -> [w533]
    tunnel: w82 -> [w534]
    tunnel: w18 -> [w529]
    stop <- w536 stop-if-true
    n148 = case shown="False" w551 {
      tunnel: w550 -> [w646 _]
      tunnel: [errorcluster {"status"=FALSE, "code"=0, "source"=""} ("error out") w651] -> w538
      tunnel: [w647 w650] -> w547
      tunnel: w546 -> [w647 _]
      tunnel: [w646 w649] -> w539
      frame False {
      }
      frame True {
        w657 = T4 12 items=["User Home"=0, "User Desktop"=1, "User Documents"=2, "User Application Data"=3, "User Preferences"=4, "User Temporary"=5, "Public Documents"=6, "Public Application Data"=7, "Public Preferences"=8, "Public Cache"=13, "System Core Libraries"=9, "System Installed Libraries"=10, "Application Files"=11, "Boot Volume Root"=12] ("system directory type")
        n149 = call <vilib>:"Get System Directory.vi"("create directory if not found? (F)"=TRUE, "system directory type"=w657) -> ("system directory"=w658:path)  [unwired: 9 in]
        n150 = Build Path(base path=w658, name or relative path="Logs\\" ("string")) -> (appended path=w654:path)
        n151 = Create Folder(path (use dialog)=w654) -> (created path=w653:path)  [unwired: 2 in, 2 out]
        n152 = Build Path(base path=w653, name or relative path="FTP File Move Record.CSV") -> (appended path=w650:path)
        n153 = Open/Create/Replace File(file path (use dialog)=w650, operation (0:open)=T9."open or create", access (0:read/write)=enum16{"read/write", "read-only", "write-only"}."read/write") -> (refnum out=w661:refnum<file>, error out=w662:errorcluster)  [unwired: 3 in, 1 out]
        n154 = Set File Position(refnum=w661, from (0:start)=enum16{"start", "end", "current"}."end", error in=w662) -> (refnum out=w649:refnum<file>, error out=w651:errorcluster)  [unwired: 1 in]
      }
    }
    n155 = local write "Status FTP move"(FALSE ("Status FTP move")) -> ()
    n156 = Get Notifier Status(notifier=w537) -> (current notification=w536:bool)  [unwired: 1 in, 4 out]
    n157 = event shown="[0] Timeout" {
      selector: _ -> [_ _]
      dyn-events: _ -> [_ _]
      timeout: 100 -> [_ _]
      tunnel: [w676 w809] -> w554
      tunnel: w553 -> [w675 w808]
      tunnel: [w674 w807] -> w545
      tunnel: w533 -> [w673 w806]
      tunnel: [w672 w805] -> w543
      tunnel: [w671 w804] -> w532
      tunnel: w539 -> [w669 w803]
      tunnel: w538 -> [w668 w802]
      tunnel: w547 -> [w667 w801]
      tunnel: "FTP Creds" -> [w666 w800]
      tunnel: w534 -> [w665 w799]
      tunnel: w529 -> [w664 w798]
      event Timeout {
        n158 = event-data() -> ()  [unwired: 1 in, 1 out]
        n159 = call "Timing 5min after 5min before.vi"() -> ("Mid Hour"=w670:bool)  [unwired: 5 in]
        n160 = case shown="True" w670 {
          tunnel: [w678 w693] -> w676
          tunnel: w675 -> [w680 w692]
          tunnel: [w680 w691] -> w674
          tunnel: w673 -> [w679 w690]
          tunnel: [w679 w689] -> w672
          tunnel: [w677 w688] -> w671
          tunnel: w669 -> [w678 w686]
          tunnel: w668 -> [w677 w685]
          tunnel: w667 -> [_ w684]
          tunnel: w666 -> [_ w683]
          tunnel: w665 -> [_ w682]
          tunnel: w664 -> [_ w681]
          frame False {
          }
          frame True {
            n161 = call "Elapsed Time2"() -> ("Time has Elapsed"=w687:bool)  [unwired: 12 in, 7 out]
            n162 = case shown="True" w687 {
              tunnel: [w694 w710] -> w693
              tunnel: w692 -> [w697 w709]
              tunnel: [w697 w708] -> w691
              tunnel: w690 -> [w696 w707]
              tunnel: [w696 w706] -> w689
              tunnel: [w695 w705] -> w688
              tunnel: w686 -> [w694 w703]
              tunnel: w685 -> [w695 w702]
              tunnel: w684 -> [_ w701]
              tunnel: w683 -> [_ w700]
              tunnel: w682 -> [_ w699]
              tunnel: w681 -> [_ w698]
              frame False {
              }
              frame True {
                n163 = stacked-sequence {
                  seq-local: [w719 _] -> [_ w737]
                  seq-local: [w718 _] -> [_ w736]
                  tunnel: [_ w740] -> w710
                  tunnel: w709 -> [w720 _]
                  tunnel: [_ w738] -> w708
                  tunnel: w707 -> [w717 w733]
                  tunnel: [_ w731] -> w706
                  tunnel: [_ w730] -> w705
                  tunnel: w703 -> [_ w729]
                  tunnel: w702 -> [w716 _]
                  tunnel: w701 -> [_ _]
                  tunnel: w700 -> [_ w728]
                  tunnel: w699 -> [_ w727]
                  tunnel: w698 -> [w713 w726]
                  frame #0 {
                    n164 = Merge Errors(w717, w716) -> (w712:errorcluster)
                    n165 = List Folder(path=w713, pattern="*.ZIP", error in=w712) -> (filenames=w714:string[], error out=w711:errorcluster)  [unwired: 1 in, 2 out]
                    n166 = for {
                      tunnel: w720 -> [w725]
                      tunnel: [w724] -> w719
                      tunnel: [w723] -> w718
                      tunnel: w714 -> [w722] mode=indexing
                      tunnel: w711 -> [w721]
                      n167 = Enqueue Element(queue=w725, element=w722, error in (no error)=w721) -> (queue out=w723:refnum<queue>, error out=w724:errorcluster)  [unwired: 1 in, 1 out]
                    }
                  }
                  frame #1 {
                    n168 = Get Queue Status(queue=w736, error in (no error)=w733) -> (queue out=w735:refnum<queue>, error out=w732:errorcluster, # elements in queue=w734:i32)  [unwired: 1 in, 5 out]
                    n169 = local read "Archive Location"() -> (w739:path)
                    n170 = for {
                      N: w734 -> [_]
                      tunnel: [w759] -> w740
                      tunnel: w737 -> [w758]
                      tunnel: w739 -> [w744]
                      tunnel: w735 -> [w747]
                      tunnel: [w755] -> w738
                      tunnel: [w757] -> w730
                      tunnel: w732 -> [w746]
                      tunnel: [w752] -> w731
                      tunnel: w729 -> [w751]
                      tunnel: w728 -> [w750]
                      tunnel: w727 -> [w748]
                      tunnel: w726 -> [w743]
                      n171 = Get Notifier Status(notifier=w748) -> (current notification=w745:bool)  [unwired: 1 in, 4 out]
                      n172 = Dequeue Element(queue=w747, timeout in ms (-1)=5, error in (no error)=w746) -> (queue out=w756:refnum<queue>, element=w741:string, error out=w753:errorcluster)  [unwired: 1 out]
                      n173 = call "FTP Move_Status_Errors.vi"("Archived Path dir"=w743, "FTP input cluster"=w750, "Queue elements"=w741) -> ("concatenated string of Error"=w742:string, "ReQue element  errored"=w749:bool)  [unwired: 7 in]
                      n174 = case shown="False" w745 {
                        tunnel: [w773 w792] -> w759
                        tunnel: w758 -> [w772 w791]
                        tunnel: [w771 w791] -> w757
                        tunnel: w756 -> [w770 w796]
                        tunnel: [w769 w795] -> w755
                        tunnel: w753 -> [w768 w794]
                        tunnel: [w767 w793] -> w752
                        tunnel: w751 -> [w766 w792]
                        tunnel: w742 -> [w765 _]
                        tunnel: w749 -> [w764 _]
                        tunnel: w741 -> [w763 _]
                        tunnel: w744 -> [w762 _]
                        tunnel: w743 -> [w761 _]
                        tunnel: w741 -> [w760 _]
                        frame False {
                          n175 = case shown="False" w764 {
                            tunnel: w770 -> [w775 w787]
                            tunnel: w763 -> [_ _]
                            tunnel: [w775 w787] -> w769
                            tunnel: w768 -> [w774 w786]
                            tunnel: [w774 w786] -> w767
                            tunnel: w762 -> [_ w781]
                            tunnel: w761 -> [_ w780]
                            tunnel: w760 -> [_ w776]
                            frame False {
                            }
                            frame True {
                              n176 = Build Path(base path=w781, name or relative path="ZIPS\\") -> (appended path=w785:path)
                              n177 = call <vilib>:"Check if File or Folder Exists.vi"("path"=w785) -> ("file or folder exists?"=w784:bool, "dup path"=w783:path)  [unwired: 8 in, 1 out]
                              n178 = Build Path(base path=w780, name or relative path=w776) -> (appended path=w779:path)
                              n179 = case shown="False" w784 {
                                tunnel: w783 -> [w789 w790]
                                tunnel: [w788 w790] -> w777
                                frame False {
                                n180 = Create Folder(path (use dialog)=w789) -> (created path=w788:path)  [unwired: 2 in, 2 out]
                                }
                                frame True {
                                }
                              }
                              n181 = Build Path(base path=w777, name or relative path=w776) -> (appended path=w778:path)
                              n182 = Move(source path=w779, 10:w778) -> ()  [unwired: 3 in, 3 out]
                            }
                          }
                          n183 = Write to Text File(file (use dialog)=w766, text=w765, error in=w772) -> (refnum out=w773:refnum<file>, error out=w771:errorcluster)  [unwired: 1 in, 1 out]
                        }
                        frame True {
                          n184 = Flush Queue(queue=w796, error in (no error)=w794) -> (queue out=w795:refnum<queue>, error out=w793:errorcluster)  [unwired: 1 out]
                        }
                      }
                    }
                  }
                }
                n185 = local write "Status FTP move"(TRUE ("Status FTP move")) -> ()
              }
            }
          }
        }
      }
      event "Manual FTP": Value Change {
        n186 = event-data() -> ()  [unwired: 1 in, 1 out]
        n187 = stacked-sequence {
          seq-local: [w818 _] -> [_ w836]
          seq-local: [w817 _] -> [_ w835]
          tunnel: [_ w839] -> w809
          tunnel: w808 -> [w819 _]
          tunnel: [_ w837] -> w807
          tunnel: w806 -> [w816 w832]
          tunnel: [_ w830] -> w805
          tunnel: [_ w829] -> w804
          tunnel: w803 -> [_ w828]
          tunnel: w802 -> [w815 _]
          tunnel: w801 -> [_ _]
          tunnel: w800 -> [_ w827]
          tunnel: w799 -> [_ w826]
          tunnel: w798 -> [w812 w825]
          frame #0 {
            n188 = Merge Errors(w816, w815) -> (w811:errorcluster)
            n189 = List Folder(path=w812, pattern="*.ZIP", error in=w811) -> (filenames=w813:string[], error out=w810:errorcluster)  [unwired: 1 in, 2 out]
            n190 = for {
              tunnel: w819 -> [w824]
              tunnel: [w823] -> w818
              tunnel: [w822] -> w817
              tunnel: w813 -> [w821] mode=indexing
              tunnel: w810 -> [w820]
              n191 = Enqueue Element(queue=w824, element=w821, error in (no error)=w820) -> (queue out=w822:refnum<queue>, error out=w823:errorcluster)  [unwired: 1 in, 1 out]
            }
          }
          frame #1 {
            n192 = Get Queue Status(queue=w835, error in (no error)=w832) -> (queue out=w834:refnum<queue>, error out=w831:errorcluster, # elements in queue=w833:i32)  [unwired: 1 in, 5 out]
            n193 = local read "Archive Location"() -> (w838:path)
            n194 = for {
              N: w833 -> [_]
              tunnel: [w858] -> w839
              tunnel: w836 -> [w857]
              tunnel: w838 -> [w843]
              tunnel: w834 -> [w846]
              tunnel: [w854] -> w837
              tunnel: [w856] -> w829
              tunnel: w831 -> [w845]
              tunnel: [w851] -> w830
              tunnel: w828 -> [w850]
              tunnel: w827 -> [w849]
              tunnel: w826 -> [w847]
              tunnel: w825 -> [w842]
              n195 = Get Notifier Status(notifier=w847) -> (current notification=w844:bool)  [unwired: 1 in, 4 out]
              n196 = Dequeue Element(queue=w846, timeout in ms (-1)=5, error in (no error)=w845) -> (queue out=w855:refnum<queue>, element=w840:string, error out=w852:errorcluster)  [unwired: 1 out]
              n197 = call "FTP Move_Status_Errors.vi"("Archived Path dir"=w842, "FTP input cluster"=w849, "Queue elements"=w840) -> ("concatenated string of Error"=w841:string, "ReQue element  errored"=w848:bool)  [unwired: 7 in]
              n198 = case shown="False" w844 {
                tunnel: [w872 w895] -> w858
                tunnel: w857 -> [w871 w894]
                tunnel: [w870 w894] -> w856
                tunnel: w855 -> [w869 w899]
                tunnel: [w868 w898] -> w854
                tunnel: w852 -> [w867 w897]
                tunnel: [w866 w896] -> w851
                tunnel: w850 -> [w865 w895]
                tunnel: w841 -> [w864 _]
                tunnel: w848 -> [w863 _]
                tunnel: w840 -> [w862 _]
                tunnel: w843 -> [w861 _]
                tunnel: w842 -> [w860 _]
                tunnel: w840 -> [w859 _]
                frame False {
                  n199 = case shown="True" w863 {
                    tunnel: w869 -> [w878 w890]
                    tunnel: w862 -> [w877 _]
                    tunnel: [w876 w890] -> w868
                    tunnel: w867 -> [w874 w889]
                    tunnel: [w873 w889] -> w866
                    tunnel: w861 -> [_ w884]
                    tunnel: w860 -> [_ w883]
                    tunnel: w859 -> [_ w879]
                    frame False {
                      n200 = Enqueue Element(queue=w878, element=w877, timeout in ms (-1)=5, error in (no error)=w874) -> (queue out=w876:refnum<queue>, error out=w873:errorcluster)  [unwired: 1 out]
                    }
                    frame True {
                      n201 = Build Path(base path=w884, name or relative path="ZIPS\\") -> (appended path=w888:path)
                      n202 = call <vilib>:"Check if File or Folder Exists.vi"("path"=w888) -> ("file or folder exists?"=w887:bool, "dup path"=w886:path)  [unwired: 8 in, 1 out]
                      n203 = Build Path(base path=w883, name or relative path=w879) -> (appended path=w882:path)
                      n204 = case shown="False" w887 {
                        tunnel: w886 -> [w892 w893]
                        tunnel: [w891 w893] -> w880
                        frame False {
                          n205 = Create Folder(path (use dialog)=w892) -> (created path=w891:path)  [unwired: 2 in, 2 out]
                        }
                        frame True {
                        }
                      }
                      n206 = Build Path(base path=w880, name or relative path=w879) -> (appended path=w881:path)
                      n207 = Move(source path=w882, 10:w881) -> ()  [unwired: 3 in, 3 out]
                    }
                  }
                  n208 = Write to Text File(file (use dialog)=w865, text=w864, error in=w871) -> (refnum out=w872:refnum<file>, error out=w870:errorcluster)  [unwired: 1 in, 1 out]
                }
                frame True {
                  n209 = Flush Queue(queue=w899, error in (no error)=w897) -> (queue out=w898:refnum<queue>, error out=w896:errorcluster)  [unwired: 1 out]
                }
              }
            }
          }
        }
        n210 = local write "Status FTP move"(TRUE ("Status FTP move")) -> ()
      }
    }
    n211 = Unbundle By Name("FTP Creds") -> ("Comp File Size"=w542:bool, "SITE ID"=w540:string)
    n212 = case shown="True" w542 {
      tunnel: w545 -> [w575 w583]
      tunnel: [w575 w582] -> w544
      tunnel: w543 -> [w574 w580]
      tunnel: [w574 w581] -> w530
      tunnel: "FTP Creds" -> [_ w579]
      tunnel: w540 -> [_ w577]
      tunnel: w529 -> [_ w576]
      frame False {
      }
      frame True {
        n213 = call "True at one time of day.vi"("Time stamp from INI (only will use time Not date)"="Time DaY") -> ("Time Until Next Scan (H)"=→"Elapsed Time (H)":dbl, "Time has Elapsed"=w584:bool)  [unwired: 8 in, 1 out]
        n214 = case shown="True" w584 {
          tunnel: w583 -> [w587 w609]
          tunnel: [w587 w611] -> w582
          tunnel: [w586 w610] -> w581
          tunnel: w580 -> [w586 w608]
          tunnel: w579 -> [_ w613]
          tunnel: w577 -> [_ w605]
          tunnel: w576 -> [_ w590]
          frame False {
          }
          frame True {
            w601 = "\r\n"
            n215 = local read "Archive Location"() -> (w591:path)
            n216 = Build Path(base path=w591, name or relative path="ZIPS\\") -> (appended path=w592:path)
            n217 = call <vilib>:"Check if File or Folder Exists.vi"("path"=w592) -> ("file or folder exists?"=w593:bool, "dup path"=w594:path)  [unwired: 8 in, 1 out]
            n218 = case shown="True" w593 {
              tunnel: w594 -> [w615 w616]
              tunnel: [w614 w616] -> w589
              frame False {
                n219 = Create Folder(path (use dialog)=w615) -> (created path=w614:path)  [unwired: 2 in, 2 out]
              }
              frame True {
              }
            }
            n220 = call "Compare file size of FTP to Dir on local Machine.vi"("File Pattern (*.CSV .ddf)"="*.ZIP", "Local Path to compare file sizes to FTP"=w589, "FTP Creds"=w613) -> ("Equal File Sizes"=w607:cluster{"name":string, "Equal File size":bool}[])  [unwired: 7 in, 1 out]
            n221 = for {
              tunnel: [w629] -> w611
              tunnel: [w628] -> w610
              tunnel: w609 -> [w626]
              tunnel: w608 -> [w627]
              tunnel: w607 -> [w625] mode=indexing
              tunnel: [w622] -> w604 mode=indexing
              shift-right: [w620] -> w606
              shift-left: 0 -> [w619]
              tunnel: w590 -> [w618]
              tunnel: w589 -> [w617]
              n222 = Unbundle By Name(w625) -> ("Equal File size"=w624:bool, "name"=w623:string)
              n223 = case shown="False" w624 {
                tunnel: [w638 w642] -> w629
                tunnel: [w637 w641] -> w628
                tunnel: w627 -> [w636 w641]
                tunnel: w626 -> [w635 w642]
                tunnel: w623 -> [w631 _]
                tunnel: [1 0] -> w621
                tunnel: [w631 ""] -> w622
                tunnel: w618 -> [w633 _]
                tunnel: w617 -> [w630 _]
                frame False {
                  n224 = Build Path(base path=w630, name or relative path=w631) -> (appended path=w632:path)
                  n225 = Copy(10:w633, 11:w632) -> ()  [unwired: 3 in, 3 out]
                  n226 = Enqueue Element(queue=w635, element=w631, error in (no error)=w636) -> (queue out=w638:refnum<queue>, error out=w637:errorcluster)  [unwired: 1 in, 1 out]
                }
                frame True {
                }
              }
              n227 = Add(x=w619, y=w621) -> (x+y=w620:i32)
            }
            n228 = local read "Email Notification"() -> (w596:T3)
            n229 = local read "recipients"() -> (w599:string[])
            n230 = Concatenate Strings("FTP VS DIR File sizes are different at Site ID: " ("string"), w605) -> (w598:string)
            n231 = Concatenate Strings(w598, w601, "These files have been re-queued for FTP move agian, check to make sure files are up to date and moving correctly.\nFiles of issue are listed below.\n\nLIST:" ("string"), w601, w604) -> (w597:string)
            n232 = Greater Than 0?(x=w606) -> (x > 0?=w600:bool)
            n233 = call "Send Email Notification.vi"("Send Email Notification"=w600, "Mail Creds"=w596, "message"=w597, "Email Subject"=w598, "recipients"=w599) -> ()  [unwired: 7 in]
          }
        }
      }
    }
    n234 = case shown="No Error" w532 {
      selector: w532 -> [w556 _]
      tunnel: [w556 errorcluster {"status"=FALSE, "code"=0, "source"=""} ("error IO")] -> w531
      frame No Error {
      }
      frame Error {
        n235 = local read "FTP Creds"() -> (w560:T2)
        n236 = Unbundle By Name(w560) -> ("SITE ID"=w559:string)
        n237 = local read "Email Notification"() -> (w562:T3)
        n238 = local read "recipients"() -> (w563:string[])
        n239 = Concatenate Strings("The Software was unable to write to the FTP Log at site ID: " ("Email Subject"), w559) -> (w557:string)
        n240 = call "Send Email Notification.vi"("Send Email Notification"=TRUE, "Mail Creds"=w562, "message"=w557, "Email Subject"=w557, "recipients"=w563) -> ()  [unwired: 7 in]
      }
    }
    n241 = Unbundle By Name(w538) -> ("status"=w549:bool)
    n242 = case shown="False" w549 {
      tunnel: [FALSE ("create directory if not found? (F)") TRUE ("create directory if not found? (F)")] -> w548
      frame False {
      }
      frame True {
        n243 = One Button Dialog(message="The File \"FTP FILE MOVE RECORD.CSV\" is open.\nPlease close the file before continuing.\n\nThis file is the log of past FTP movement and is needed by the software to maintain a history of already moved file. Please do not move or delete this file. This will result in unwanted actions by the software in attempt to send all files back up to the ftp again.\n") -> ()  [unwired: 1 in, 1 out]
      }
    }
    n244 = case shown="No Error" w530 {
      selector: w530 -> [w565 _]
      tunnel: [w565 errorcluster {"status"=FALSE, "code"=0, "source"=""} ("error IO")] -> w535
      frame No Error {
      }
      frame Error {
        n245 = local read "Email Notification"() -> (w571:T3)
        n246 = local read "recipients"() -> (w572:string[])
        n247 = local read "FTP Creds"() -> (w569:T2)
        n248 = Unbundle By Name(w569) -> ("SITE ID"=w568:string)
        n249 = Concatenate Strings("There was an Error with the FTP scan and Move at Site ID: " ("Email Subject"), w568) -> (w566:string)
        n250 = call "Send Email Notification.vi"("Send Email Notification"=TRUE, "Mail Creds"=w571, "message"=w566, "Email Subject"=w566, "recipients"=w572) -> ()  [unwired: 7 in]
      }
    }
  }
  n251 = while {
    shift-right: [w901] -> w125
    shift-left: w126 -> [w918]
    shift-right: [w906] -> w120
    shift-left: w82 -> [w909]
    tunnel: [w916] -> w240
    tunnel: [w915] -> w239
    tunnel: [w914] -> w238
    tunnel: w18 -> [w900]
    stop <- w907 stop-if-true
    n252 = local read "FTP Creds"() -> (w913:T2)
    n253 = local write "Status File move"(FALSE ("Status File move")) -> ()
    n254 = Equal?(x="Archive Location 2", y=path "") -> (x = y?=w926:bool)
    n255 = call <vilib>:"Check if File or Folder Exists.vi"("path"="Archive Location 2") -> ("file or folder exists?"=w925:bool, "dup path"=w921:path)  [unwired: 8 in, 1 out]
    n256 = Compound Arithmetic op=AND(w925, invert w926) -> (w922:bool)
    n257 = event shown="[0] Timeout" {
      selector: _ -> [_ _ _]
      dyn-events: _ -> [_ _ _]
      timeout: 30 -> [_ _ _]
      tunnel: w913 -> [w957 w1085 _]
      tunnel: w922 -> [w956 w1084 _]
      tunnel: w921 -> [w955 w1083 w1174]
      tunnel: "Archive Location" -> [w954 w1082 w1175]
      tunnel: "Rats Location" -> [w953 w1081 w1176]
      tunnel: w918 -> [w952 w1080 w1172]
      tunnel: [w951 w1079 w1171] -> w904
      tunnel: [w950 w1078 w1176] -> w916
      tunnel: [w949 w1077 w1175] -> w915
      tunnel: [w948 w1076 w1174] -> w914
      tunnel: w900 -> [w946 w1075 _]
      event Timeout {
        n258 = event-data() -> ()  [unwired: 1 in, 1 out]
        n259 = call "Timing 5min after 5min before.vi"() -> ("Mid Hour"=w947:bool)  [unwired: 5 in]
        n260 = case shown="True" w947 {
          tunnel: w953 -> [w961 w973]
          tunnel: w954 -> [w960 w972]
          tunnel: w955 -> [w959 w971]
          tunnel: w956 -> [_ w970]
          tunnel: w957 -> [_ w968]
          tunnel: [w961 w967] -> w950
          tunnel: [w960 w966] -> w949
          tunnel: [w959 w965] -> w948
          tunnel: w952 -> [w958 w964]
          tunnel: [w958 w963] -> w951
          tunnel: w946 -> [_ w962]
          frame False {
          }
          frame True {
            n261 = call "Elapsed Time"() -> ("Time has Elapsed"=w969:bool)  [unwired: 12 in, 7 out]
            n262 = case shown="True" w969 {
              tunnel: w973 -> [w977 w989]
              tunnel: w972 -> [w976 w988]
              tunnel: w971 -> [w975 w987]
              tunnel: w970 -> [_ w986]
              tunnel: w968 -> [_ w985]
              tunnel: [w977 w980] -> w967
              tunnel: [w976 w979] -> w966
              tunnel: [w975 w978] -> w965
              tunnel: w964 -> [w974 w984]
              tunnel: [w974 w983] -> w963
              tunnel: w962 -> [_ w981]
              frame False {
              }
              frame True {
                n263 = stacked-sequence {
                  seq-local: [_ w1003 _ _ _] -> [_ _ w1016 _ _]
                  seq-local: [w997 _ _ _ _] -> [_ w1009 _ _ _]
                  seq-local: [w996 _ _ _ _] -> [_ w1002 _ _ _]
                  seq-local: [_ w1006 _ _ _] -> [_ _ w1015 _ _]
                  seq-local: [_ _ w1014 _ _] -> [_ _ _ w1050 _]
                  tunnel: w989 -> [w993 _ _ _ w1073]
                  tunnel: w988 -> [_ _ _ w1033 w1072]
                  tunnel: w987 -> [w994 _ _ _ w1071]
                  tunnel: w986 -> [w995 _ _ _ _]
                  tunnel: w985 -> [w992 _ _ _ _]
                  tunnel: w984 -> [w991 _ _ _ _]
                  tunnel: [_ _ _ w1050 _] -> w983
                  tunnel: w981 -> [w990 w1001 w1013 w1030 _]
                  tunnel: [_ _ _ _ w1073] -> w980
                  tunnel: [_ _ _ _ w1072] -> w979
                  tunnel: [_ _ _ _ w1071] -> w978
                  frame #0 {
                    n264 = Unbundle By Name(w992) -> ("Use ATL"=w1000:bool)
                    n265 = Select(t="*.ATL" ("pattern"), s=w1000, f="dont use the ALT files" ("pattern")) -> (s? t:f=w997:string)
                    n266 = call "File Move (incoming to Archive).vi"("Rats Location"=w993, "Archive Location"=w990, "Archive Location 2"=w994, "Archive 2 valid path"=w995, "error IO 2"=w991, "pattern"=w997) -> ("error IO"=w996:errorcluster)  [unwired: 9 in]
                  }
                  frame #1 {
                    n267 = call "Directory to list File compare.vi"("2nd File Type(s)(*.txt *.CSV)"="*.zip", "1st File Type(s)(*.txt *.CSV)"=w1009, "error in (no error)"=w1002, "2nd Directory (Zip)"=w1001, "1st Directory (RATS)"=w1001) -> ("error out"=w1008:errorcluster, "Unmanaged Files"=w1005:string[])  [unwired: 4 in, 1 out]
                    n268 = call "Directory to list File compare.vi"("2nd File Type(s)(*.txt *.CSV)"="*.zip", "1st File Type(s)(*.txt *.CSV)"="*.RAT" ("2nd File Type(s)(*.txt *.CSV)"), "error in (no error)"=w1002, "2nd Directory (Zip)"=w1001, "1st Directory (RATS)"=w1001) -> ("error out"=w1007:errorcluster, "Unmanaged Files"=w1004:string[])  [unwired: 4 in, 1 out]
                    n269 = Insert Into Array(array=w1005, new element=w1004) -> (w1003:string[])  [unwired: 1 in]
                    n270 = Merge Errors(w1008, w1007) -> (w1006:errorcluster)
                  }
                  frame #2 {
                    n271 = for {
                      tunnel: w1016 -> [w1018] mode=indexing
                      tunnel: w1013 -> [w1017]
                      shift-right: [w1023] -> w1014
                      shift-left: w1015 -> [w1024]
                      n272 = String To Path(string=w1018) -> (path=w1025:path)
                      n273 = Build Path(base path=w1017, name or relative path=w1018) -> (appended path=w1021:path)
                      n274 = Concatenate Strings(w1018, ".Zip" ("name or relative path")) -> (w1019:string)
                      n275 = Build Path(base path=w1017, name or relative path=w1019) -> (appended path=w1022:path)
                      n276 = call <vilib>:"New Zip File.vi"("error in (no error)"=w1024, "target"=w1022) -> ("error out"=w1026:errorcluster, "zip file out"=w1029:i64)  [unwired: 3 in, 1 out]
                      n277 = call <vilib>:"Add File to Zip.vi"("error in (no error)"=w1026, "destination path in zip"=w1025, "source file path"=w1021, "zip file in"=w1029) -> ("error out"=w1028:errorcluster, "zip file out"=w1027:i64)  [unwired: 6 in]
                      n278 = call <vilib>:"Close Zip File.vi"("error in (no error)"=w1028, "zip file in"=w1027) -> ("error out"=w1023:errorcluster)  [unwired: 5 in]
                    }
                  }
                  frame #3 {
                    n279 = Build Path(base path=w1033, name or relative path="RATS\\") -> (appended path=w1045:path)
                    n280 = Build Path(base path=w1033, name or relative path="ATLS\\") -> (appended path=w1038:path)
                    n281 = call <vilib>:"Check if File or Folder Exists.vi"("path"=w1045) -> ("file or folder exists?"=w1044:bool, "dup path"=w1043:path)  [unwired: 8 in, 1 out]
                    n282 = call <vilib>:"Check if File or Folder Exists.vi"("path"=w1038) -> ("file or folder exists?"=w1039:bool, "dup path"=w1040:path)  [unwired: 8 in, 1 out]
                    n283 = case shown="True" w1044 {
                      tunnel: w1043 -> [w1062 w1063]
                      tunnel: [w1061 w1063] -> w1031
                      frame False {
                        n284 = Create Folder(path (use dialog)=w1062) -> (created path=w1061:path)  [unwired: 2 in, 2 out]
                      }
                      frame True {
                      }
                    }
                    n285 = case shown="True" w1039 {
                      tunnel: w1040 -> [w1052 w1053]
                      tunnel: [w1051 w1053] -> w1032
                      frame False {
                        n286 = Create Folder(path (use dialog)=w1052) -> (created path=w1051:path)  [unwired: 2 in, 2 out]
                      }
                      frame True {
                      }
                    }
                    n287 = List Folder(path=w1030, pattern="*.RAT") -> (path out=w1048:path, filenames=w1049:string[], error out=w1047:errorcluster)  [unwired: 2 in, 1 out]
                    n288 = List Folder(path=w1030, pattern="*.ATL") -> (path out=w1035:path, filenames=w1034:string[], error out=w1036:errorcluster)  [unwired: 2 in, 1 out]
                    n289 = for {
                      tunnel: w1049 -> [w1069] mode=indexing
                      tunnel: w1048 -> [w1070]
                      tunnel: w1047 -> [w1066]
                      tunnel: [w1065] -> _
                      tunnel: w1031 -> [w1064]
                      n290 = Build Path(base path=w1070, name or relative path=w1069) -> (appended path=w1068:path)
                      n291 = Move(source path=w1068, error in=w1066, 9:TRUE ("overwrite (F)"), 10:w1064) -> (error out=w1065:errorcluster)  [unwired: 1 in, 2 out]
                    }
                    n292 = for {
                      tunnel: w1034 -> [w1059] mode=indexing
                      tunnel: w1035 -> [w1060]
                      tunnel: w1036 -> [w1056]
                      tunnel: [w1055] -> _
                      tunnel: w1032 -> [w1054]
                      n293 = Build Path(base path=w1060, name or relative path=w1059) -> (appended path=w1058:path)
                      n294 = Move(source path=w1058, error in=w1056, 9:TRUE ("overwrite (F)"), 10:w1054) -> (error out=w1055:errorcluster)  [unwired: 1 in, 2 out]
                    }
                  }
                  frame #4 {
                  }
                }
                n295 = local write "Status File move"(TRUE ("Status File move")) -> ()
              }
            }
          }
        }
      }
      event "Manual Archive": Value Change {
        n296 = event-data() -> ()  [unwired: 1 in, 5 out]
        n297 = stacked-sequence {
          seq-local: [_ w1099 _ _ _] -> [_ _ w1112 _ _]
          seq-local: [w1093 _ _ _ _] -> [_ w1105 _ _ _]
          seq-local: [w1092 _ _ _ _] -> [_ w1098 _ _ _]
          seq-local: [_ w1102 _ _ _] -> [_ _ w1111 _ _]
          seq-local: [_ _ w1110 _ _] -> [_ _ _ w1146 _]
          tunnel: w1081 -> [w1089 _ _ _ w1170]
          tunnel: w1082 -> [_ _ _ w1129 w1169]
          tunnel: w1083 -> [w1090 _ _ _ w1168]
          tunnel: w1084 -> [w1091 _ _ _ _]
          tunnel: w1085 -> [w1088 _ _ _ w1167]
          tunnel: w1080 -> [w1087 _ _ _ _]
          tunnel: [_ _ _ w1146 _] -> w1079
          tunnel: w1075 -> [w1086 w1097 w1109 w1126 _]
          tunnel: [_ _ _ _ w1170] -> w1078
          tunnel: [_ _ _ _ w1169] -> w1077
          tunnel: [_ _ _ _ w1168] -> w1076
          tunnel: [_ _ _ _ w1167] -> _
          frame #0 {
            n298 = Unbundle By Name(w1088) -> ("Use ATL"=w1096:bool)
            n299 = Select(t="*.ATL" ("pattern"), s=w1096, f="dont use the ALT files" ("pattern")) -> (s? t:f=w1093:string)
            n300 = call "File Move (incoming to Archive).vi"("Rats Location"=w1089, "Archive Location"=w1086, "Archive Location 2"=w1090, "Archive 2 valid path"=w1091, "error IO 2"=w1087, "pattern"=w1093) -> ("error IO"=w1092:errorcluster)  [unwired: 9 in]
          }
          frame #1 {
            n301 = call "Directory to list File compare.vi"("2nd File Type(s)(*.txt *.CSV)"="*.zip", "1st File Type(s)(*.txt *.CSV)"=w1105, "error in (no error)"=w1098, "2nd Directory (Zip)"=w1097, "1st Directory (RATS)"=w1097) -> ("error out"=w1104:errorcluster, "Unmanaged Files"=w1101:string[])  [unwired: 4 in, 1 out]
            n302 = call "Directory to list File compare.vi"("2nd File Type(s)(*.txt *.CSV)"="*.zip", "1st File Type(s)(*.txt *.CSV)"="*.RAT" ("2nd File Type(s)(*.txt *.CSV)"), "error in (no error)"=w1098, "2nd Directory (Zip)"=w1097, "1st Directory (RATS)"=w1097) -> ("error out"=w1103:errorcluster, "Unmanaged Files"=w1100:string[])  [unwired: 4 in, 1 out]
            n303 = Insert Into Array(array=w1101, new element=w1100) -> (w1099:string[])  [unwired: 1 in]
            n304 = Merge Errors(w1104, w1103) -> (w1102:errorcluster)
          }
          frame #2 {
            n305 = for {
              tunnel: w1112 -> [w1114] mode=indexing
              tunnel: w1109 -> [w1113]
              shift-right: [w1119] -> w1110
              shift-left: w1111 -> [w1120]
              n306 = String To Path(string=w1114) -> (path=w1121:path)
              n307 = Build Path(base path=w1113, name or relative path=w1114) -> (appended path=w1117:path)
              n308 = Concatenate Strings(w1114, ".Zip" ("name or relative path")) -> (w1115:string)
              n309 = Build Path(base path=w1113, name or relative path=w1115) -> (appended path=w1118:path)
              n310 = call <vilib>:"New Zip File.vi"("error in (no error)"=w1120, "target"=w1118) -> ("error out"=w1122:errorcluster, "zip file out"=w1125:i64)  [unwired: 3 in, 1 out]
              n311 = call <vilib>:"Add File to Zip.vi"("error in (no error)"=w1122, "destination path in zip"=w1121, "source file path"=w1117, "zip file in"=w1125) -> ("error out"=w1124:errorcluster, "zip file out"=w1123:i64)  [unwired: 6 in]
              n312 = call <vilib>:"Close Zip File.vi"("error in (no error)"=w1124, "zip file in"=w1123) -> ("error out"=w1119:errorcluster)  [unwired: 5 in]
            }
          }
          frame #3 {
            n313 = Build Path(base path=w1129, name or relative path="RATS\\") -> (appended path=w1141:path)
            n314 = Build Path(base path=w1129, name or relative path="ATLS\\") -> (appended path=w1134:path)
            n315 = call <vilib>:"Check if File or Folder Exists.vi"("path"=w1141) -> ("file or folder exists?"=w1140:bool, "dup path"=w1139:path)  [unwired: 8 in, 1 out]
            n316 = call <vilib>:"Check if File or Folder Exists.vi"("path"=w1134) -> ("file or folder exists?"=w1135:bool, "dup path"=w1136:path)  [unwired: 8 in, 1 out]
            n317 = case shown="False" w1140 {
              tunnel: w1139 -> [w1158 w1159]
              tunnel: [w1157 w1159] -> w1127
              frame False {
                n318 = Create Folder(path (use dialog)=w1158) -> (created path=w1157:path)  [unwired: 2 in, 2 out]
              }
              frame True {
              }
            }
            n319 = case shown="False" w1135 {
              tunnel: w1136 -> [w1148 w1149]
              tunnel: [w1147 w1149] -> w1128
              frame False {
                n320 = Create Folder(path (use dialog)=w1148) -> (created path=w1147:path)  [unwired: 2 in, 2 out]
              }
              frame True {
              }
            }
            n321 = List Folder(path=w1126, pattern="*.RAT") -> (path out=w1144:path, filenames=w1145:string[], error out=w1143:errorcluster)  [unwired: 2 in, 1 out]
            n322 = List Folder(path=w1126, pattern="*.ATL") -> (path out=w1131:path, filenames=w1130:string[], error out=w1132:errorcluster)  [unwired: 2 in, 1 out]
            n323 = for {
              tunnel: w1145 -> [w1165] mode=indexing
              tunnel: w1144 -> [w1166]
              tunnel: w1143 -> [w1162]
              tunnel: [w1161] -> _
              tunnel: w1127 -> [w1160]
              n324 = Build Path(base path=w1166, name or relative path=w1165) -> (appended path=w1164:path)
              n325 = Move(source path=w1164, error in=w1162, 9:TRUE ("overwrite (F)"), 10:w1160) -> (error out=w1161:errorcluster)  [unwired: 1 in, 2 out]
            }
            n326 = for {
              tunnel: w1130 -> [w1155] mode=indexing
              tunnel: w1131 -> [w1156]
              tunnel: w1132 -> [w1152]
              tunnel: [w1151] -> _
              tunnel: w1128 -> [w1150]
              n327 = Build Path(base path=w1156, name or relative path=w1155) -> (appended path=w1154:path)
              n328 = Move(source path=w1154, error in=w1152, 9:TRUE ("overwrite (F)"), 10:w1150) -> (error out=w1151:errorcluster)  [unwired: 1 in, 2 out]
            }
          }
          frame #4 {
          }
        }
        n329 = local write "Status File move"(TRUE ("Status File move")) -> ()
      }
      event Menu Selection (User) {
        n330 = event-data() -> ("ItemTag"=w1177:string)  [unwired: 1 in]
        n331 = case shown="\"Exit\"" w1177 {
          tunnel: [errorcluster {"status"=FALSE, "code"=0, "source"=""} ("error out") w1179 errorcluster {"status"=FALSE, "code"=0, "source"=""} ("error out")] -> w1173
          frame "Null", Default {
          }
          frame "Exit" {
            n332 = Obtain Notifier(name (unnamed)="Shutdown", notification data type=TRUE) -> (notifier out=w1182:refnum<notifier>, error out=w1184:errorcluster)  [unwired: 2 in, 1 out]
            n333 = Send Notification(notification=TRUE, notifier=w1182, error in (no error)=w1184) -> (error out=w1179:errorcluster)  [unwired: 1 out]
          }
          frame "NAF" {
            n334 = call "About.vi"() -> ()  [unwired: 12 in]
          }
        }
        n335 = Merge Errors(w1173, w1172) -> (w1171:errorcluster)
      }
    }
    n336 = case shown="False" "ShutDown" {
      tunnel: [FALSE ("Status File move") w944] -> w910
      frame False {
      }
      frame True {
        n337 = Two Button Dialog(message="Are you sure you want to shut down NODE ARCHIVE & FTP? This will end all file management of the Archive directories and FTP file movement until the software is restarted.\nIf the Archiving In Progress, or the FTP In Progress is lit the software will shut down as soon as the process is done.", 2:"Shutdown" ("T button name (\"OK\")")) -> (T button?=w944:bool)  [unwired: 1 in]
      }
    }
    n338 = case shown="False" w910 {
      tunnel: w909 -> [w928 w931]
      tunnel: [w928 w930] -> w908
      tunnel: [errorcluster {"status"=FALSE, "code"=0, "source"=""} ("error out") w929] -> w905
      frame False {
      }
      frame True {
        n339 = Send Notification(notification=TRUE, notifier=w931) -> (notifier out=w930:refnum<notifier>, error out=w929:errorcluster)  [unwired: 1 in]
      }
    }
    n340 = Get Notifier Status(notifier=w908, error in (no error)=w905) -> (notifier out=w906:refnum<notifier>, current notification=w907:bool, error out=w903:errorcluster)  [unwired: 2 out]
    n341 = Merge Errors(w904, w903) -> (w902:errorcluster)
    n342 = case shown="No Error" w902 {
      selector: w902 -> [w933 _]
      tunnel: [w933 errorcluster {"status"=FALSE, "code"=0, "source"=""} ("error IO")] -> w901
      frame No Error {
      }
      frame Error {
        n343 = local read "FTP Creds"() -> (w937:T2)
        n344 = Unbundle By Name(w937) -> ("SITE ID"=w936:string)
        n345 = local read "Email Notification"() -> (w939:T3)
        n346 = local read "recipients"() -> (w940:string[])
        n347 = Concatenate Strings("Archiving and Zipping  at Site: " ("Email Subject"), w936) -> (w934:string)
        n348 = call "Send Email Notification.vi"("Send Email Notification"=TRUE, "Mail Creds"=w939, "message"=w934, "Email Subject"=w934, "recipients"=w940) -> ()  [unwired: 7 in]
      }
    }
  }
  n349 = call <vilib>:"Get System Directory.vi"("create directory if not found? (F)"=TRUE, "system directory type"=w169) -> ("system directory"=w168:path)  [unwired: 9 in]
  n350 = Build Path(base path=w168, name or relative path="Logs\\" ("string")) -> (appended path=w172:path)
  n351 = Create Folder(path (use dialog)=w172) -> (created path=w173:path)  [unwired: 2 in, 2 out]
  n352 = Build Path(base path=w173, name or relative path="Node FTP and STATS.INI") -> (appended path=w167:path)
  n353 = call <vilib>:"Open Config Data.vi"("create file if necessary (T)"=TRUE, "configuration file path"=w167) -> ("error out"=w255:errorcluster, "refnum"=w256:T6)  [unwired: 7 in, 1 out]
  n354 = call-poly <vilib>:"Write Key.vi"("section"=w262, "error in (no error)"=w255, "value"=w240, "key"="Rat Locations" ("name or relative path"), "refnum"=w256) -> ("error out"=w258:errorcluster, "refnum out"=w257:T6)  [unwired: 4 in, 1 out]
  n355 = call-poly <vilib>:"Write Key.vi"("section"=w262, "error in (no error)"=w258, "value"=w239, "key"="Archive" ("name or relative path"), "refnum"=w257) -> ("error out"=w260:errorcluster, "refnum out"=w259:T6)  [unwired: 4 in, 1 out]
  n356 = call-poly <vilib>:"Write Key.vi"("section"=w262, "error in (no error)"=w260, "value"=w238, "key"="Archive 2" ("name or relative path"), "refnum"=w259) -> ("error out"=w266:errorcluster, "refnum out"=w272:T6)  [unwired: 4 in, 1 out]
  n357 = Unbundle By Name(w189) -> ("Host"=w253:string, "UserName"=w252:string, "PassWord"=w251:string, "FTP File Path"=w250:string, "FTP Timeout (S)"=w249:i32, "Use ATL"=w248:bool, "Comp File Size"=w211:bool, "SITE ID"=w190:string, "Active or Passive"=w4:bool, "ASCII or Binary"=w3:bool)
  n358 = call-poly <vilib>:"Write Key.vi"("section"=w7, "error in (no error)"=w266, "value"=w253, "key"="Host" ("name or relative path"), "refnum"=w272) -> ("error out"=w267:errorcluster, "refnum out"=w273:T6)  [unwired: 4 in, 1 out]
  n359 = call-poly <vilib>:"Write Key.vi"("section"=w7, "error in (no error)"=w267, "value"=w252, "key"="UserName" ("name or relative path"), "refnum"=w273) -> ("error out"=w268:errorcluster, "refnum out"=w274:T6)  [unwired: 4 in, 1 out]
  n360 = call-poly <vilib>:"Write Key.vi"("section"=w7, "error in (no error)"=w268, "value"=w251, "key"="Password" ("name or relative path"), "refnum"=w274) -> ("error out"=w269:errorcluster, "refnum out"=w275:T6)  [unwired: 4 in, 1 out]
  n361 = Merge Errors(w182, w141, w140) -> (w181:errorcluster)
  n362 = call-poly <vilib>:"Write Key.vi"("section"=w7, "error in (no error)"=w269, "value"=w250, "key"="FTP File Path" ("name or relative path"), "refnum"=w275) -> ("error out"=w270:errorcluster, "refnum out"=w276:T6)  [unwired: 4 in, 1 out]
  n363 = call-poly <vilib>:"Write Key.vi"("section"=w7, "error in (no error)"=w270, "value"=w249, "key"="FTP Timeout" ("name or relative path"), "refnum"=w276) -> ("error out"=w271:errorcluster, "refnum out"=w277:T6)  [unwired: 4 in, 1 out]
  n364 = call-poly <vilib>:"Write Key.vi"("section"=w7, "error in (no error)"=w271, "value"=w248, "key"="Archive Zip .ATL" ("name or relative path"), "refnum"=w277) -> ("error out"=w11:errorcluster, "refnum out"=w10:T6)  [unwired: 4 in, 1 out]
  n365 = call-poly <vilib>:"Write Key.vi"("section"=w7, "error in (no error)"=w11, "value"=w4, "key"="Active or Passive (Active = True)" ("name or relative path"), "refnum"=w10) -> ("error out"=w9:errorcluster, "refnum out"=w8:T6)  [unwired: 4 in, 1 out]
  n366 = call-poly <vilib>:"Write Key.vi"("section"=w7, "error in (no error)"=w9, "value"=w3, "key"="Binary or ASCII (ASCII = True) " ("name or relative path"), "refnum"=w8) -> ("error out"=w1:errorcluster, "refnum out"=w2:T6)  [unwired: 4 in, 1 out]
  n367 = call-poly <vilib>:"Write Key.vi"("section"=w215, "error in (no error)"=w1, "value"=w210, "key"="File size Compare (FTP to DIR)" ("name or relative path"), "refnum"=w2) -> ("error out"=w217:errorcluster, "refnum out"=w216:T6)  [unwired: 4 in, 1 out]
  n368 = call-poly <vilib>:"Write Key.vi"("section"=w215, "error in (no error)"=w217, "value"=w211, "key"="Use File size Compare (FTP to DIR)" ("name or relative path"), "refnum"=w216) -> ("error out"=w194:errorcluster, "refnum out"=w193:T6)  [unwired: 4 in, 1 out]
  n369 = Release Queue(queue=w218, error in (no error)=w115) -> (error out=w116:errorcluster)  [unwired: 1 in, 2 out]
  n370 = Close File(refnum=w237, error in=w114) -> (error out=w117:errorcluster)  [unwired: 1 out]
  n371 = Unbundle By Name(w97) -> ("AddressNode 1"=w86:string, "AddressNode2"=w85:string, "Addresshost"=w84:string)
  n372 = call-poly <vilib>:"Write Key.vi"("section"="SITE" ("name or relative path"), "error in (no error)"=w194, "value"=w190, "key"="Site ID" ("name or relative path"), "refnum"=w193) -> ("error out"=w89:errorcluster, "refnum out"=w90:T6)  [unwired: 4 in, 1 out]
  n373 = Merge Errors(w116, w117, w181) -> (w232:errorcluster)
  n374 = call-poly <vilib>:"Write Key.vi"("section"=w94, "error in (no error)"=w89, "value"=w86, "key"="Node 1" ("Mail Server"), "refnum"=w90) -> ("error out"=w88:errorcluster, "refnum out"=w95:T6)  [unwired: 4 in, 1 out]
  n375 = call-poly <vilib>:"Write Key.vi"("section"=w94, "error in (no error)"=w88, "value"=w85, "key"="Node 2" ("Mail Server"), "refnum"=w95) -> ("error out"=w87:errorcluster, "refnum out"=w96:T6)  [unwired: 4 in, 1 out]
  n376 = call-poly <vilib>:"Write Key.vi"("section"=w94, "error in (no error)"=w87, "value"=w84, "key"="FTP Host" ("Mail Server"), "refnum"=w96) -> ("error out"=w38:errorcluster, "refnum out"=w39:T6)  [unwired: 4 in, 1 out]
  n377 = Unbundle By Name(w35) -> ("Mail Server"=w34:string, "Return Address"=w33:string, "Email User Name"=w32:string, "Password"=w31:string)
  n378 = call-poly <vilib>:"Write Key.vi"("section"=w26, "error in (no error)"=w38, "value"=w34, "key"="Mail Server" ("Mail Server"), "refnum"=w39) -> ("error out"=w44:errorcluster, "refnum out"=w45:T6)  [unwired: 4 in, 1 out]
  n379 = call-poly <vilib>:"Write Key.vi"("section"=w26, "error in (no error)"=w44, "value"=w33, "key"="Return Address" ("Return Address"), "refnum"=w45) -> ("error out"=w46:errorcluster, "refnum out"=w49:T6)  [unwired: 4 in, 1 out]
  n380 = call-poly <vilib>:"Write Key.vi"("section"=w26, "error in (no error)"=w46, "value"=w32, "key"="User Name" ("Email User Name"), "refnum"=w49) -> ("error out"=w47:errorcluster, "refnum out"=w48:T6)  [unwired: 4 in, 1 out]
  n381 = call-poly <vilib>:"Write Key.vi"("section"=w26, "error in (no error)"=w47, "value"=w31, "key"="Password" ("Password"), "refnum"=w48) -> ("error out"=w52:errorcluster, "refnum out"=w51:T6)  [unwired: 4 in, 1 out]
  n382 = Array To Spreadsheet String(delimiter (Tab)=",", array=w30, 3:"%s" ("format string")) -> (spreadsheet string=w27:string)
  n383 = call-poly <vilib>:"Write Key.vi"("section"=w26, "error in (no error)"=w52, "value"=w27, "key"="Email_Recipients" ("Password"), "refnum"=w51) -> ("error out"=w36:errorcluster, "refnum out"=w37:T6)  [unwired: 4 in, 1 out]
  n384 = call <vilib>:"Close Config Data.vi"("error in (no error)"=w36, "write file if changed (T)"=TRUE, "refnum"=w37) -> ("error out"=w162:errorcluster)  [unwired: 7 in, 1 out]
  n385 = case shown="Error" w162 {
    selector: w162 -> [w1186 _]
    tunnel: [w1186 errorcluster {"status"=FALSE, "code"=0, "source"=""} ("error IO")] -> w83
    frame No Error {
    }
    frame Error {
      w1190 = T7 4 items=["no dialog", "OK message", "continue or stop message", "OK message + warnings", "continue/stop + warnings"] ("type of dialog (OK msg:1)")
      n386 = call <vilib>:"Simple Error Handler.vi"("error code (no error:0)"=5002, "error source (\" \")"="Writing values to the INI File" ("error source (\" \")"), "type of dialog (OK msg:1)"=w1190) -> ()  [unwired: 2 in, 5 out]
    }
  }
  n387 = Merge Errors(w83, w125, w232) -> (w121:errorcluster)
  n388 = Release Notifier(notifier=w120, force destroy? (F)=TRUE, error in (no error)=w121) -> (error out=w123:errorcluster)  [unwired: 2 out]
  n389 = call <vilib>:"Clear Errors.vi"("error in (no error)"=w123) -> ("error out"=w122:errorcluster)  [unwired: 6 in]
  n390 = property class="App"(error in=w122) -> (error out=w124:errorcluster, "App.Kind"=w233:T10)  [unwired: 1 in, 1 out]
  n391 = case shown="\"Run Time System\"" w233 {
    tunnel: w124 -> [_ _ _ _ _ _ _]
    frame "invalid app kind", Default {
    }
    frame "Development System" {
    }
    frame "Run Time System" {
      n392 = Quit LabVIEW() -> ()  [unwired: 1 in]
    }
    frame "Student Edition" {
    }
    frame "Embedded LabVIEW" {
    }
    frame "Evaluation" {
    }
    frame "Custom" {
    }
  }
  "Status File move" <- FALSE ("Status File move")
  "Status FTP move" <- FALSE ("Status FTP move")
